vi "Core_Chem_User_Interface_v1.0.vi"() -> ()   [LabVIEW 2014]
uses:
  <vilib>/dex/Stream Element Allocation Mode.ctl
  C:/Program Files (x86)/National Instruments/LabVIEW 2014/examples/Data Communication/Network Streams/Simple Network Streams/support/Network Stream Command.ctl
  <vilib>/Platform/TimedLoop/XDataNode/timing_clust.ctl
  <vilib>/Platform/TimedLoop/XDataNode/nitl_modes.ctl
  <vilib>/Platform/TimedLoop/XDataNode/wakeup.ctl
  <vilib>/Utility/tcp.llb/UDP Multicast Read-Only Open.vi
  <vilib>/platform/TimedLoop/XDataNode/XDataNode.xnode
  <vilib>/Platform/TimedLoop/XDataNode/XDNodeRunTimeDep.lvlib
  <vilib>/FTP/NI_FTP.lvlib
panel:
  out "Create folder error out 2":errorcluster
  out "Network to cRIO live status":bool
  out "Create folder error out":errorcluster
  out "PRTUDP\nerror out":errorcluster
  in  "Confirm Flight Number":bool
  out "PRTAFT_UDP_In":string
  out "TWBOZO01":string
  out "CABOZO01":string
  out "TEIOZO01":string
  out "CHTSOO01":string
  out "CHFGGA01":string
  out "AL52CO01":string
  in  "Flight Number":string
  in  "Tab Control":T1(tab)
  out "MFM":dbl(graph)
  in  "name":string="239.1.4.6"
  in  "Port":u16=50001
  out "FGGA":string
  out "CO":string
  out "Ozone":string
  out "Cabin Ozone":string
  out "Ambient Ozone":string
  out "SO2":string
  out "CO Concentration":dbl(graph)
  out "Fluorsecence Cell Pressure":dbl(graph)
  out "Monochromater Flow":dbl(graph)
  out "Lamp Flow Controller":dbl(graph)
  in  "CO UDP Time Offset":i32=1
  out "CO2 Pressure\nDelivery (PSIA)":dbl(slide) scale=0.0..100.0
  out "CO CAL Status":bool
  out "Std\nContent (barG)":dbl(slide) scale=0.0..220.0
  out "N2\nContent (barG)":dbl(slide) scale=0.0..220.0
  out "CO2\nContent (barG)":dbl(slide) scale=0.0..170.0
  in  "CO CAL":bool
  in  "CO Vacuum (eV7)":bool
  out "CO Event error out":errorcluster
  out "CO command sender error out":errorcluster
  out "CO Zero":T2(array[cluster])
  out "CO Sensitivity":T3(array[cluster])
  in  "Ozone V6":bool
  out "TEI49C Sample Flow B":dbl(graph)
  out "TEi49C Concentration":dbl(graph)
  out "TEI49C Sample Flow A":dbl(graph)
  out "Ozone Event error out":errorcluster
  out "Ozone command sender error out":errorcluster
  out "Ozone Zeroing\nTime Remain (sec)":u32
  in  "Ozone Zeroing":bool
  in  "Ozone UDP Time Offset":i32=1
  in  "FGGA Pump":bool
  in  "FGGA Shutdown":bool
  in  "V1":bool
  in  "V2":bool
  in  "MFC_1\nSLPM Value":dbl
  in  "V3":bool
  in  "V4":bool
  in  "FGGA Restart":bool
  out "MFC1 Cal Flow":dbl(graph)
  out "Cell temperature":dbl(graph)
  out "Cell pressure":dbl(graph)
  out "CO2 Dry":dbl(graph)
  out "CH4 Dry":dbl(graph)
  out "H2O":dbl(graph)
  out "CO2":dbl(graph)
  out "CH4":dbl(graph)
  in  "Flush High Tank":bool
  in  "Flush Low Tank":bool
  in  "Flush Target Tank":bool
  out "Flush High Tank\nTime Remain (sec)":u32
  out "Flush Low Tank\nTime Remain (sec)":u32
  out "Flush Target Tank\nTime Remain (sec)":u32
  in  "High Cal":bool
  out "High Cal\nFlush Time Remain (sec)":u32
  out "High Cal\nCal Time Remain (sec)":u32
  in  "Low Cal":bool
  in  "Target Cal":bool
  in  "Span Cal":bool
  out "Low Cal\nFlush Time Remain (sec)":u32
  out "Low Cal\nCal Time Remain (sec)":u32
  out "Target Cal\nFlush Time Remain (sec)":u32
  out "Target Cal\nCal Time Remain (sec)":u32
  in  "MFC_1 User Set Value":dbl=3.0
  out "FGGA command sender error out":errorcluster
  out "FGGA Event Error out":errorcluster
  in  "FGGA UDP Time Offset":i32=1
  in  "FGGA pump\nsync to WoW":bool
  out "WoW Flag":string="0"
  in  "Inst_alm_thresh":i32=220
  in  "3hr_alm_thresh":i32=80
  in  "Simulate Inst Conc":i32
  in  "Simulate 3hr Average Conc":dbl
  in  "Simulate 2B Conc":bool
  out "2B Ozone concentration":dbl(graph)
  out "2B Ozone flow rate":dbl(graph)
  out "2BOzone Event error out":errorcluster
  out "2BOzone command sender error out":errorcluster
  in  "Ambient = OFF\nCabin = ON":bool
  in  "V9":bool
  in  "V8":bool
  in  "SO2 V6":bool
  in  "MFC_2\nSLPM Value":dbl
  in  "MFC_3\nSLPM Value":dbl=2.0
  in  "Simulate STEL Conc":dbl
  in  "Simulate TWA Conc":dbl
  in  "SO2 Offset":dbl
  in  "SO2 Slope":dbl=1.0
  in  "10mins STEL Limit":i32=700
  in  "8hr TWA Limit":i32=490
  in  "Simulate Conc":bool
  out "TEI43i MFC2 Cal Flow":dbl(graph)
  out "TEI43i MFC3 Sample Flow":dbl(graph)
  out "TEi43C Concentration":dbl(graph)
  out "TEI43C Sample Flow":dbl(graph)
  out "SO2 Event error out":errorcluster
  out "SO2 command sender error out":errorcluster
  in  "SO2 Flush":bool
  in  "SO2 CAL":bool
  in  "MFC_2 User Set Value":dbl=2.5
  in  "MFC_3 User Set Value":dbl=2.0
  out "SO2 Flush\nTime Remain (sec)":u32
  in  "SO2 Zeroing":bool
  out "SO2 Zeroing\nTime Remain (sec)":u32
  out "SO2 CAL\nTime Remain (sec)":u32
  in  "SO2 UDP Time Offset":i32=1
  in  "cRIO File IO Stop\n(USB Flash Drive Unmount)":bool
  in  "FTP ASCII Files to Local":bool
  in  "Transfer FGGA Files":bool
  out "File List":string[](array[string])
  out "FGGA File Transfer Error out":errorcluster
  out "Move to FM Error out":errorcluster
  out "USB Disk Space Used %":dbl(slide) scale=0.0..100.0
  out "PTP Sync":bool
  out "CPU Total %":dbl(graph)
  # "ch4\nco2\nh2o\npress_torr\ntemp_c\nfit_flag\nrda_usec\nrdb_usec\nch4_dry\nco2_dry\nMFC_1_absolute_pressure\nMFC_1_temperature\nMFC_1volumetic_flow\nMFC_1mass_flow\nMFC_1set_point\nV1\nV2\nV3\nV4\nrestart_FGGA\nFGGA_Pump\nCAL_MFC_1Set_Value"
  # "conc\ntemp\npress\nflow\nthreehr_oz\nInst_alarm\nthreehr_alarm"
  # "conc\ntemp\npress\nflow"
  # "concentration\npmt_volt\nlamp_volt\nlamp_intens\ninternal_temper\nreact_temper\nreact_press\nflow\nflags\nten_min_so2\neight_hr_so2\nten_min_so2_alm\neight_hr_so2_alm\nMFC_2absolute_pressure\nMFC_2temperature\nMFC_2volumetic_flow\nMFC_2mass_flow\nMFC_2set_point\nMFC_3_absolute_pressure\nMFC_3_temperature\nMFC_3volumetic_flow\nMFC_3mass_flow\nMFC_3set_point\nV6\nV8\nV9\nMFC2_Set_Value\nMFC3_Set_Value"
  # "conc\nbenchtemp\npress\ncellAint\ncellBint\nFlowA\nFlowB\nlamptemp\nflag\nV6"
  # "conc\ncounts\nsens\nzero\nlampflow\nlamptemp\nmonoflow\nmonotemp\nmonopress\ncellpress\ncalpress\ntemppmt\ncalconc\nerr\ncal_counter\nerr_counter\nCO_vacuum_status\nIn_Cal\nALEG1_press_delivery\nALREG1_press_content\nALREG2_press_content\nALREG3_press_content"
  # "DIRECT CONTROL"
  # "DIRECT CONTROLS"
  # "DIRECT CONTROLS"
  # "TEi43c"
  # "TEi43i"
  # "DIRECT CONTROLS"
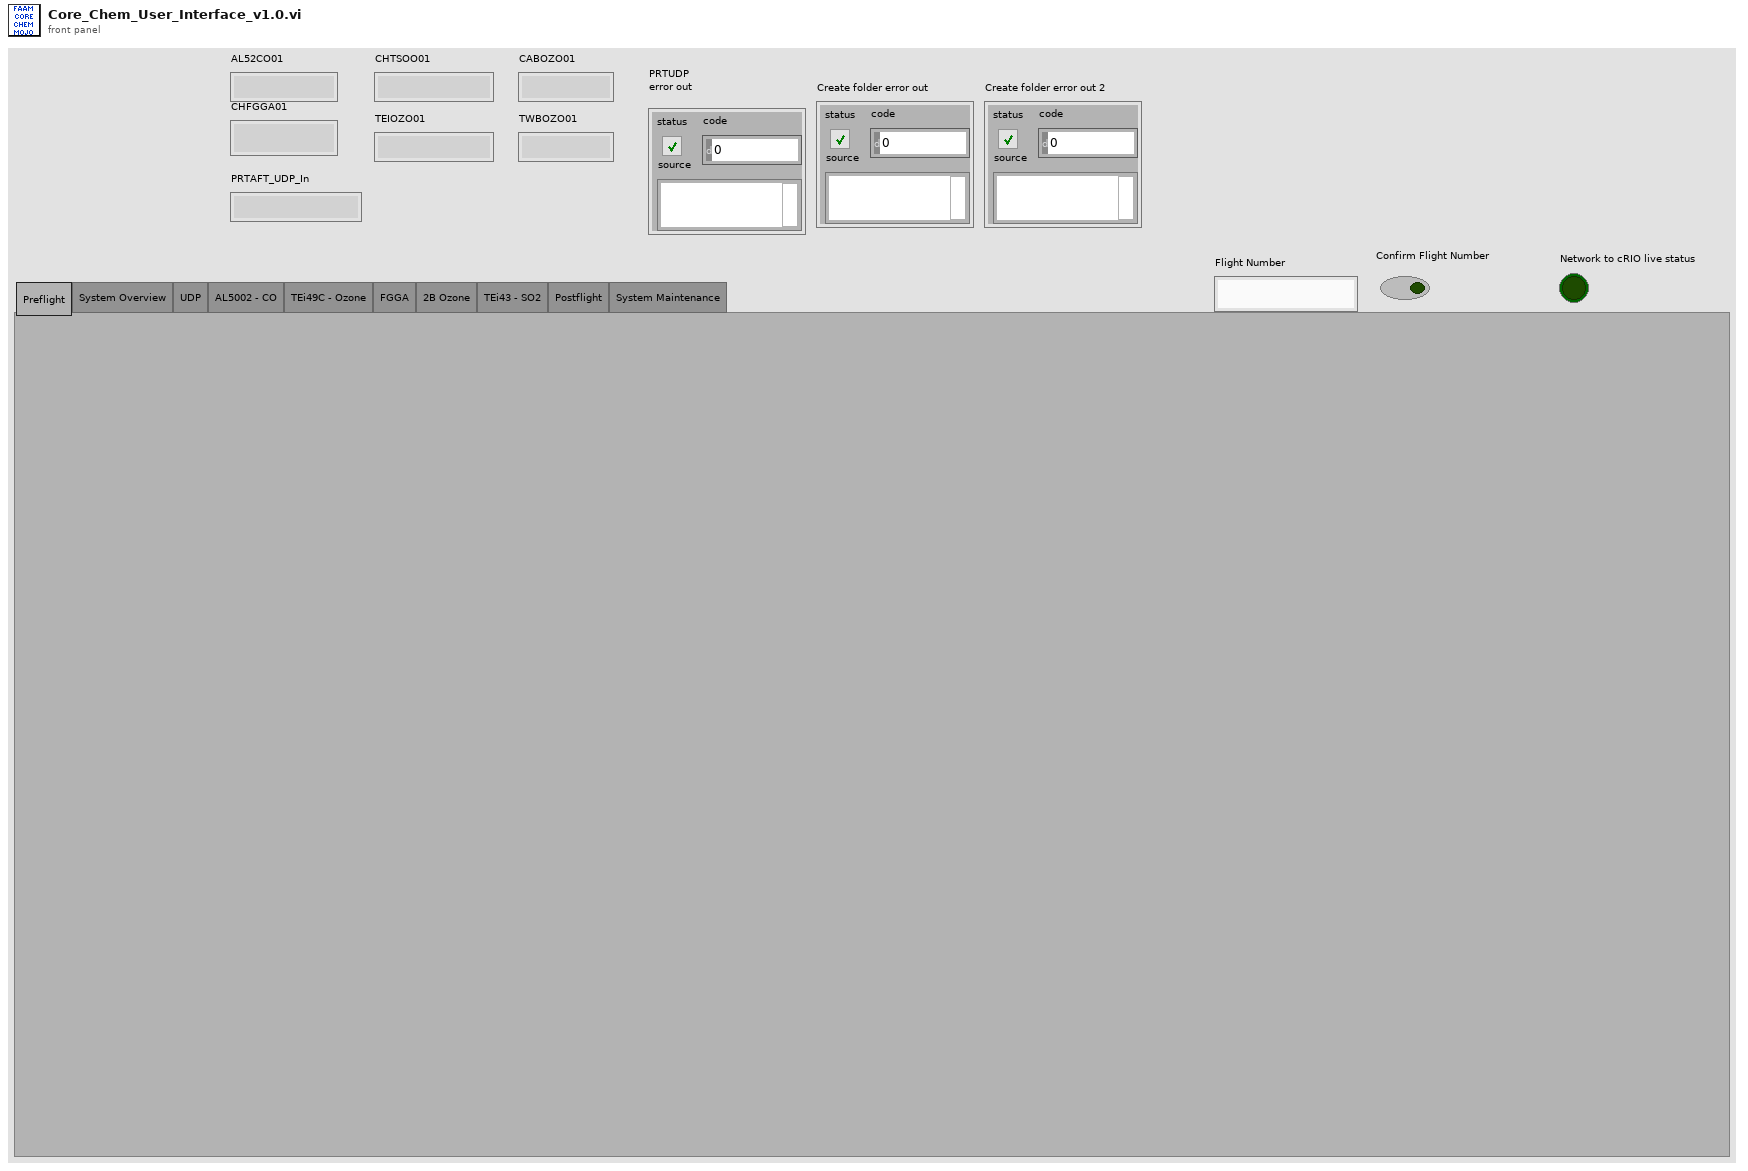
[diagram p1: front panel]
types:
  T1 = enum32{"Preflight", "System Overview", "UDP", "AL5002 - CO", "TEi49C - Ozone", "FGGA", "2B Ozone", "TEi43 - SO2", "Postflight", "System Maintenance"}
  T2 = cluster{"time stamp":timestamp, "CO Offset":dbl}[]
  T3 = cluster{"time stamp":timestamp, "CO Sensitivity":dbl}[]
  T4 = typedef "Network Stream Command.ctl" = cluster{"Message":string, "Message Data":variant}
  T5 = typedef "Stream Element Allocation Mode.ctl" = u32
  T6 = typedef "XDNodeRunTimeDep.lvlib/timing_clust.ctl" = cluster{"Expected End [f-1]":u64, "Actual End [f-1]":u64, "Finished Late? [f-1]":bool, "Expected End [i-1]":u64, "Actual End [i-1]":u64, "Finished Late? [i-1]":bool, "Expected Start [i]":u64, "Actual Start [i]":u64, "Expected Start [f]":u64, "Actual Start [f]":u64, "Source Name":string, "Structure Name":string, "Period":i64, "Deadline":i64, "Offset":i64, "Start":i64, "Priority":i32, "Timeout":i32, "Mode":T7, "Wakeup Reason":T8, "Error":errorcluster, "Source Type":string, "Secondary Source Type":string, "Global End Time":u64, "Global Start Time":u64, "Frame Duration":u64, "Iteration Duration":u64, "Assigned CPU":i32, "I/O Scan Engine Mode":u32}
  T7 = typedef "XDNodeRunTimeDep.lvlib/nitl_modes.ctl" = enum32{"No Change", "Process missed periods, maintain original phase", "Discard missed periods, maintain original phase", "Process missed periods, ignore original phase", "Discard missed periods, ignore original phase"}
  T8 = typedef "XDNodeRunTimeDep.lvlib/wakeup.ctl" = enum32{"Normal", "Aborted", "Asynchronous wakeup", "Timing source error", "Timed loop error", "Timeout"}
  T9 = typedef "NI_FTP.lvlib/FTP Session.ctl" = refnum<k5>
  T10 = typedef "NI_FTP.lvlib/FTP File Info.ctl" = cluster{"type":enum16{"unknown", "file", "dir", "link"}, "permissions":string, "owner":string, "group":string, "size":i32, "date":string, "name":string, "link name":string}
  T11 = cluster{"Message":string, "Message 2":string, "Message 3":string}
  T12 = cluster{"Message":string, "Message 2":string, "Message 3":string, "Message 4":string}
  T13 = cluster{"Message":string, "Message 3":string, "Message 4":string}
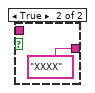
[diagram p7: hidden frame]
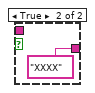
[diagram p8: hidden frame]
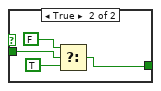
[diagram p9: hidden frame]
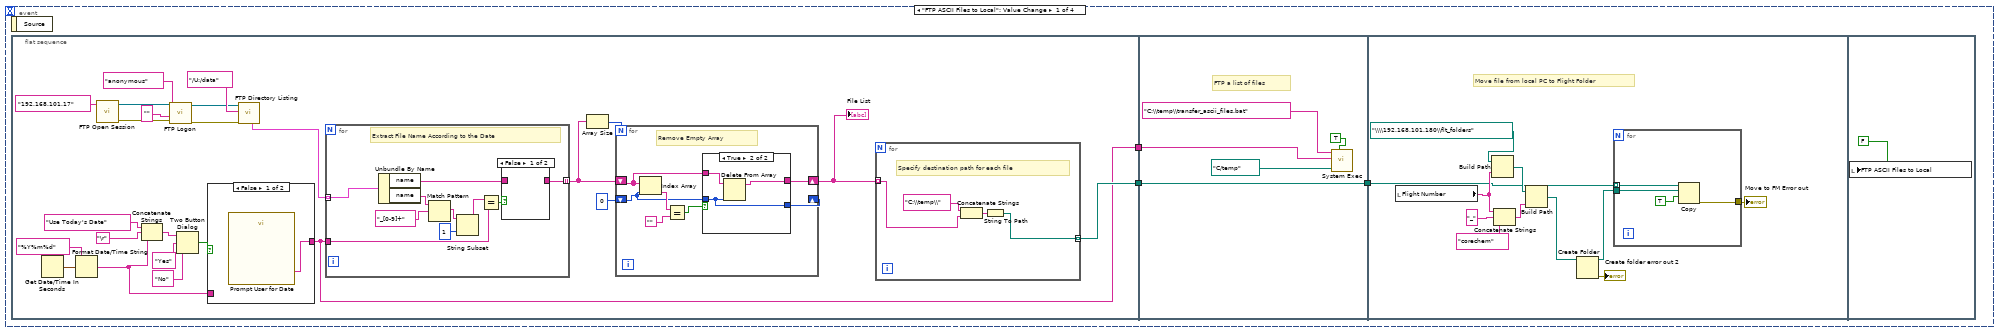
[diagram p12: hidden frame]
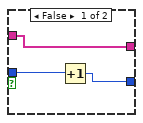
[diagram p14: hidden frame]
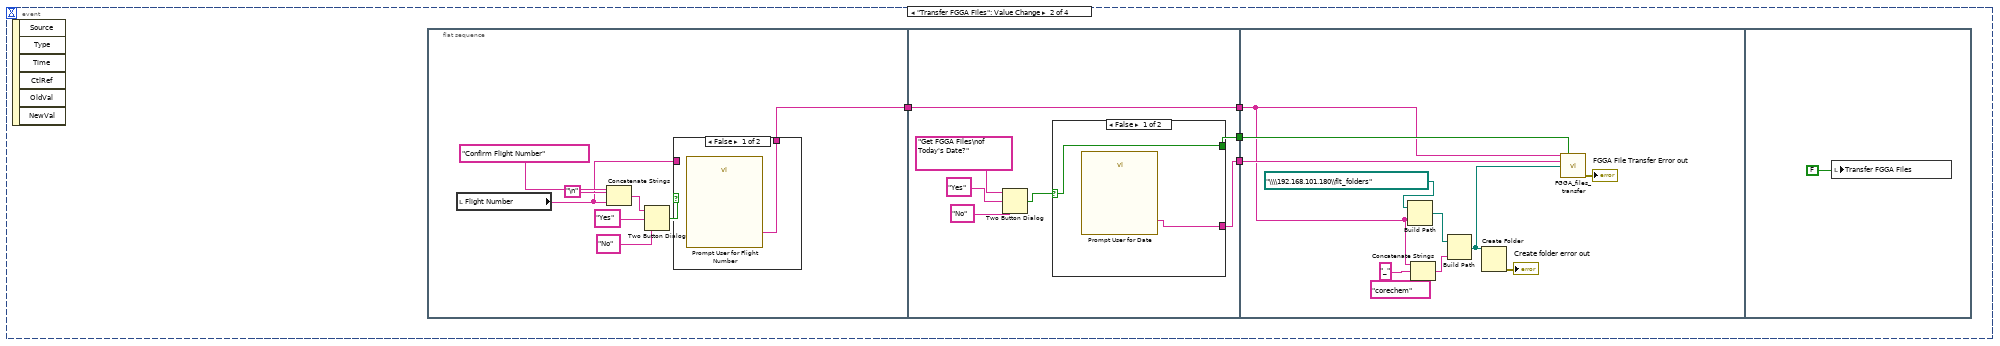
[diagram p16: hidden frame]
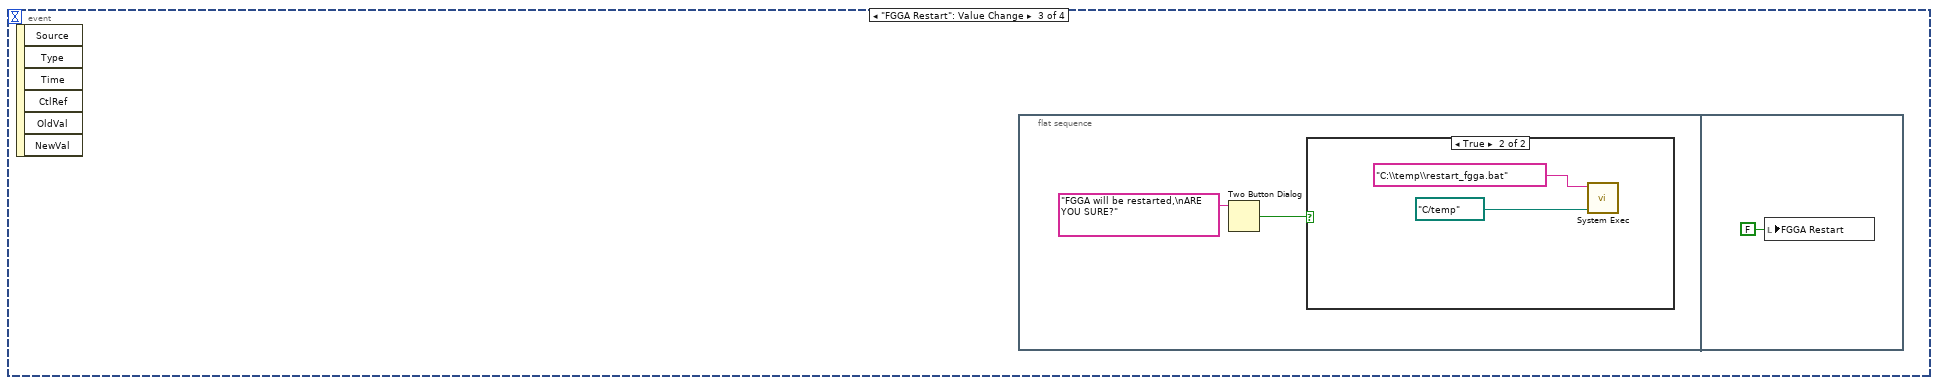
[diagram p19: hidden frame]
diagram:
  w4 = "XXXX"
  w7 = 0
  w8 = 0.0
  w14 = T4 {"Message"="", "Message Data"=variant} ("Message Cluster")
  w20 = T5 0 items=["allocate as needed", "pre-allocate"] ("element allocation mode")
  w26 = T4 {"Message"="", "Message Data"=variant} ("Message Cluster")
  w32 = T5 0 items=["allocate as needed", "pre-allocate"] ("element allocation mode")
  w37 = T4 {"Message"="", "Message Data"=variant} ("Message Cluster")
  w43 = T5 0 items=["allocate as needed", "pre-allocate"] ("element allocation mode")
  w53 = T5 0 items=["allocate as needed", "pre-allocate"] ("element allocation mode")
  w55 = T4 {"Message"="", "Message Data"=variant} ("Message Cluster")
  w62 = T5 0 items=["allocate as needed", "pre-allocate"] ("element allocation mode")
  w64 = T4 {"Message"="", "Message Data"=variant} ("Message Cluster")
  n1 = local write "cRIO File IO Stop\n(USB Flash Drive Unmount)"(FALSE ("Stop File Write")) -> ()
  n2 = local write "Flight Number"(w4) -> ()
  n3 = while {
    shift-right: [w68] -> _
    shift-left: w4 -> [w67]
    stop <- FALSE stop-if-true
    n4 = Not Equal?(x=w67, y="Flight Number") -> (x != y?=w70:bool)
    n5 = case shown="True" w70 {
      tunnel: [w73 w74] -> w68
      tunnel: "Flight Number" -> [_ w74]
      tunnel: w67 -> [w73 _]
      frame False {
      }
      frame True {
        n6 = One Button Dialog(message="Flight Number changed,\nPress flight number button to confirm") -> ()  [unwired: 1 in, 1 out]
      }
    }
    n7 = Wait (ms)(milliseconds to wait=u32 1000) -> ()  [unwired: 1 out]
  }
  n8 = while {
    stop <- w78 stop-if-true
    n9 = String To IP(1:"239.1.4.6" ("name")) -> (0:w85:u32)
    n10 = node-c288() -> (w87:T6)  [unwired: 4 in]
    n11 = call-poly <vilib>:"UDP Multicast Open.vi"("multicast addr"=w85, "port"=u16 50001) -> ("error out"=w81:errorcluster, "connection ID"=w82:refnum<k16>)  [unwired: 7 in, 1 out]
    n12 = timed-loop {
      tunnel: w82 -> [w99]
      tunnel: w81 -> [w98]
      timing: w87 -> [_]
      timing-out: [_] -> w86
      tunnel: [w92] -> w80
      tunnel: [w90] -> w79
      tunnel: [w88] -> w78
      stop <- w89 stop-if-true
      w88 = FALSE
      # "Extract string from port aft DLU"
      # "Get Flight Number loop"
      # "Read UDP & extract flight number and WoW flag"
      n13 = node-c288() -> ()  [unwired: 1 in, 1 out]
      n14 = UDP Read(connection ID=w99, 8:w98) -> (data out=w97:string, error out=w90:errorcluster, 3:w92:refnum<k16>)  [unwired: 2 in, 2 out]
      "PRTAFT_UDP_In" <- w97
      n15 = Match Pattern(string=w97, regular expression="$PRTAFT01") -> (after substring=w93:string)  [unwired: 1 in, 3 out]
      n16 = Not Equal?(x=w93, y="") -> (x != y?=w94:bool)
      n17 = case shown="True" w94 {
        tunnel: w93 -> [_ w112]
        frame False {
        }
        frame True {
          # "Extract flight number & WoW Flag"
          n18 = Spreadsheet String To Array(delimiter (Tab)=",", format string="%s", spreadsheet string=w112, array type (2D Dbl)=string[] []) -> (array=w106:string[])
          n19 = Index Array(array=w106, index=5) -> (element=w108:string)
          n20 = Index Array(array=w106, index=19) -> (element=w104:string)
          n21 = Equal?(x=w104, y="") -> (x = y?=w103:bool)
          n22 = Equal?(x=w108, y="") -> (x = y?=w111:bool)
          n23 = case shown="False" w111 {
            tunnel: [w119 "XXXX"] -> w109
            tunnel: w108 -> [w119 _]
            frame False {
            }
            frame True {
            }
          }
          n24 = case shown="False" w103 {
            tunnel: [w117 "XXXX"] -> w102
            tunnel: w104 -> [w117 _]
            frame False {
            }
            frame True {
            }
          }
          n25 = local write "Flight Number"(w109) -> ()
          n26 = local write "WoW Flag"(w102) -> ()
        }
      }
      n27 = Unbundle(w90) -> ("status"=w91:bool)  [unwired: 2 out]
      n28 = node-c288() -> ()  [unwired: 1 in, 1 out]
      n29 = Compound Arithmetic op=OR(w91, w88) -> (w89:bool)
    }
    n30 = Wait (ms)(milliseconds to wait=u32 1000) -> ()  [unwired: 1 out]
    n31 = node-c288(w86) -> ()  [unwired: 1 out]
    n32 = UDP Close(connection ID=w80, 8:w79) -> (error out=→"PRTUDP\nerror out":errorcluster)  [unwired: 1 out]
  }
  n33 = while {
    stop <- FALSE stop-if-true
    # "UDP Read"
    n34 = String To IP(1:"name") -> (0:w128:u32)
    n35 = call-poly <vilib>:"UDP Multicast Open.vi"("multicast addr"=w128, "port"="Port") -> ("error out"=w126:errorcluster, "connection ID"=w125:refnum<k16>)  [unwired: 7 in, 1 out]
    n36 = Wait (ms)(milliseconds to wait=u32 1000) -> ()  [unwired: 1 out]
    n37 = case shown="No Error" w126 {
      selector: w126 -> [w132 _]
      tunnel: w125 -> [w131 _]
      frame No Error {
        w130 = ""
        n38 = while {
          tunnel: w132 -> [w172]
          tunnel: w131 -> [w171]
          shift-right: [w167] -> _
          shift-left: w130 -> [w168]
          shift-right: [w158] -> _
          shift-left: w130 -> [w160]
          shift-right: [w152] -> _
          shift-left: w130 -> [w154]
          shift-right: [w146] -> _
          shift-left: w130 -> [w147]
          shift-right: [w140] -> _
          shift-left: w130 -> [w141]
          shift-right: [w133] -> _
          shift-left: w130 -> [w135]
          stop <- w170 stop-if-true
          n39 = UDP Read(connection ID=w171, 8:w172) -> (data out=w134:string, error out=w170:errorcluster)  [unwired: 2 in, 3 out]
          n40 = Match Pattern(string=w134, regular expression="$TEIOZO01,") -> (match substring=w166:string, after substring=w165:string)  [unwired: 1 in, 2 out]
          n41 = Match Pattern(string=w134, regular expression="$TWBOZO01,") -> (match substring=w144:string, after substring=w143:string)  [unwired: 1 in, 2 out]
          n42 = Match Pattern(string=w134, regular expression="$CABOZO01,") -> (match substring=w150:string, after substring=w149:string)  [unwired: 1 in, 2 out]
          n43 = Match Pattern(string=w134, regular expression="$CHTSOO01,") -> (match substring=w138:string, after substring=w137:string)  [unwired: 1 in, 2 out]
          n44 = Match Pattern(string=w134, regular expression="$CHFGGA01,") -> (match substring=w162:string, after substring=w161:string)  [unwired: 1 in, 2 out]
          n45 = Match Pattern(string=w134, regular expression="$AL52CO01,") -> (match substring=w156:string, after substring=w155:string)  [unwired: 1 in, 2 out]
          n46 = Concatenate Strings(w166, w165) -> (w164:string)
          n47 = Concatenate Strings(w144, w143) -> (w142:string)
          n48 = Concatenate Strings(w150, w149) -> (w148:string)
          n49 = Concatenate Strings(w138, w137) -> (w136:string)
          n50 = Concatenate Strings(w162, w161) -> (w159:string)
          n51 = Concatenate Strings(w156, w155) -> (w153:string)
          n52 = Replace Substring(4:w142, 5:w141) -> (1:w140:string)  [unwired: 2 in, 1 out]
          "TWBOZO01" <- w140
          n53 = Replace Substring(4:w164, 5:w168) -> (1:w167:string)  [unwired: 2 in, 1 out]
          "TEIOZO01" <- w167
          n54 = Replace Substring(4:w148, 5:w147) -> (1:w146:string)  [unwired: 2 in, 1 out]
          "CABOZO01" <- w146
          n55 = Replace Substring(4:w136, 5:w135) -> (1:w133:string)  [unwired: 2 in, 1 out]
          "CHTSOO01" <- w133
          n56 = Replace Substring(4:w153, 5:w154) -> (1:w152:string)  [unwired: 2 in, 1 out]
          "AL52CO01" <- w152
          n57 = Replace Substring(4:w159, 5:w160) -> (1:w158:string)  [unwired: 2 in, 1 out]
          "CHFGGA01" <- w158
        }
      }
      frame Error {
      }
    }
  }
  n58 = Obtain Queue(name (unnamed)="CO_Command", element data type=w64) -> (queue out=w13:refnum<queue>, error out=w58:errorcluster)  [unwired: 3 in, 1 out]
  n59 = Create Network Stream Writer Endpoint(6:w62, 7:10 ("writer buffer size"), 9:w64, 10:"//192.168.101.17/command/reader/CO" ("reader url"), 11:"/command/writer/CO" ("writer name")) -> (0:w61:errorcluster, 3:w60:refnum<k21>)  [unwired: 2 in]
  n60 = while {
    tunnel: w13 -> [w176]
    tunnel: w58 -> [w175]
    tunnel: [w173] -> _
    stop <- FALSE stop-if-true
    # "CO UI Event Handler Loop"
    n61 = event shown="[4] \"Confirm Flight Number\": Value Change" {
      selector: _ -> [_ _ _ _ _]
      dyn-events: _ -> [_ _ _ _ _]
      timeout: _ -> [_ _ _ _ _]
      tunnel: w176 -> [w183 w190 w194 w201 w208]
      tunnel: w175 -> [w182 w189 w193 w200 w207]
      tunnel: [w177 w184 w192 w199 w206] -> w173
      event "CO CAL": Value Change {
        n62 = event-data() -> ("NewVal"=w180:bool)  [unwired: 1 in]
        n63 = Bundle(cluster=T4 {"Message"="", "Message Data"=variant} ("Message Cluster"), "Message"="CO CAL", "Message Data"=w180) -> (w178:T4)
        n64 = Enqueue Element(queue=w183, element=w178, error in (no error)=w182) -> (error out=w177:errorcluster)  [unwired: 1 in, 2 out]
      }
      event "CO UDP Time Offset": Value Change {
        n65 = event-data() -> ("NewVal"=w187:i32)  [unwired: 1 in]
        n66 = Bundle(cluster=T4 {"Message"="", "Message Data"=variant} ("Message Cluster"), "Message"="UDP Time Offset", "Message Data"=w187) -> (w185:T4)
        n67 = Enqueue Element(queue=w190, element=w185, error in (no error)=w189) -> (error out=w184:errorcluster)  [unwired: 1 in, 2 out]
      }
      event "CO Vacuum (eV7)": Value Change {
        n68 = event-data() -> ("NewVal"=w191:bool)  [unwired: 1 in]
        n69 = Bundle(cluster=T4 {"Message"="", "Message Data"=variant} ("Message Cluster"), "Message"="CO Vacuum", "Message Data"=w191) -> (w195:T4)
        n70 = Enqueue Element(queue=w194, element=w195, error in (no error)=w193) -> (error out=w192:errorcluster)  [unwired: 1 in, 2 out]
      }
      event "cRIO File IO Stop\n(USB Flash Drive Unmount)": Value Change {
        n71 = event-data() -> ("NewVal"=w198:bool)  [unwired: 1 in]
        n72 = Bundle(cluster=T4 {"Message"="", "Message Data"=variant} ("Message Cluster"), "Message"="Stop File Write", "Message Data"=w198) -> (w202:T4)
        n73 = Enqueue Element(queue=w201, element=w202, error in (no error)=w200) -> (error out=w199:errorcluster)  [unwired: 1 in, 2 out]
      }
      event "Confirm Flight Number": Value Change {
        n74 = event-data() -> ()  [unwired: 1 in, 1 out]
        n75 = local read "Flight Number"() -> (w205:string)
        n76 = Bundle(cluster=T4 {"Message"="", "Message Data"=variant} ("Message Cluster"), "Message"="Flight Number", "Message Data"=w205) -> (w209:T4)
        n77 = Enqueue Element(queue=w208, element=w209, error in (no error)=w207) -> (error out=w206:errorcluster)  [unwired: 1 in, 2 out]
      }
    }
    "CO Event error out" <- w173
  }
  n78 = while {
    tunnel: w13 -> [w219]
    shift-right: [w214] -> _
    shift-left: w60 -> [w216]
    shift-right: [w212] -> w49
    shift-left: w61 -> [w218]
    tunnel: w58 -> [w213]
    stop <- w212 stop-if-true
    # "CO UI Command Sender"
    n79 = Dequeue Element(queue=w219, error in (no error)=w213) -> (element=w215:T4)  [unwired: 1 in, 3 out]
    n80 = Unbundle By Name(w215) -> ("Message"=w217:string)
    n81 = case shown="\"UDP Time Offset\"" w217 {
      tunnel: w218 -> [w220 w224 w231 w238 w245 w252]
      tunnel: w216 -> [w221 w227 w234 w241 w248 w255]
      tunnel: w215 -> [_ w226 w233 w240 w247 w254]
      tunnel: [w220 w223 w230 w237 w244 w251] -> w212
      tunnel: [w221 w222 w229 w236 w243 w250] -> w214
      frame "False", Default {
      }
      frame "CO CAL" {
        n82 = shared-variable-write(w227, w224, w226) -> (w225:refnum<k21>, w228:errorcluster)  [unwired: 1 in, 1 out]
        n83 = Flush Stream(8:w228, 11:w225) -> (0:w223:errorcluster, 3:w222:refnum<k21>)  [unwired: 2 in, 1 out]
      }
      frame "UDP Time Offset" {
        n84 = shared-variable-write(w234, w231, w233) -> (w232:refnum<k21>, w235:errorcluster)  [unwired: 1 in, 1 out]
        n85 = Flush Stream(8:w235, 11:w232) -> (0:w230:errorcluster, 3:w229:refnum<k21>)  [unwired: 2 in, 1 out]
      }
      frame "Stop File Write" {
        n86 = shared-variable-write(w241, w238, w240) -> (w239:refnum<k21>, w242:errorcluster)  [unwired: 1 in, 1 out]
        n87 = Flush Stream(8:w242, 11:w239) -> (0:w237:errorcluster, 3:w236:refnum<k21>)  [unwired: 2 in, 1 out]
      }
      frame "Flight Number" {
        n88 = shared-variable-write(w248, w245, w247) -> (w246:refnum<k21>, w249:errorcluster)  [unwired: 1 in, 1 out]
        n89 = Flush Stream(8:w249, 11:w246) -> (0:w244:errorcluster, 3:w243:refnum<k21>)  [unwired: 2 in, 1 out]
      }
      frame "CO Vacuum" {
        n90 = shared-variable-write(w255, w252, w254) -> (w253:refnum<k21>, w256:errorcluster)  [unwired: 1 in, 1 out]
        n91 = Flush Stream(8:w256, 11:w253) -> (0:w251:errorcluster, 3:w250:refnum<k21>)  [unwired: 2 in, 1 out]
      }
    }
  }
  "CO command sender error out" <- w49
  n92 = node-c288() -> (w12:T6)  [unwired: 4 in]
  n93 = Initialize Array(cluster{"time stamp":timestamp, "Y":dbl} {"time stamp"=timestamp(0 s since 1904-01-01), "Y"=0.0}, 30 ("dimension size")) -> (w9:cluster{"time stamp":timestamp, "Y":dbl}[])
  n94 = timed-loop {
    timing: w12 -> [_]
    timing-out: [_] -> w11
    stop <- _ stop-if-true
    # "PC Tasks"
    n95 = node-c288() -> ()  [unwired: 1 in, 1 out]
    n96 = event shown="[3] \"FGGA Shutdown\": Value Change" {
      selector: _ -> [_ _ _ _]
      dyn-events: _ -> [_ _ _ _]
      timeout: _ -> [_ _ _ _]
      event "FTP ASCII Files to Local": Value Change {
        n97 = event-data() -> ()  [unwired: 1 in, 1 out]
        n98 = flat-sequence {
          tunnel: [w263] -> w261
          tunnel: [w262] -> w259
          tunnel: w261 -> [w320]
          tunnel: [w320] -> w260
          tunnel: w259 -> [w316]
          tunnel: w260 -> [w325]
          frame #0 {
            n99 = Get Date/Time In Seconds() -> (seconds since 1Jan1904=w267:timestamp)
            n100 = Format Date/Time String(time format string (%c)="%Y%m%d", seconds (now)=w267) -> (date/time string=w265:string)  [unwired: 1 in]
            n101 = call <vilib>:"FTP Open Session.vi"("address"="192.168.101.17") -> ("error out"=w282:errorcluster, "ftp session"=w283:T9)  [unwired: 7 in, 2 out]
            n102 = Concatenate Strings("Use Today's Date" ("message"), "\r", w265) -> (w271:string)
            n103 = call <vilib>:"FTP Logon.vi"("error in (no error)"=w282, "password"="", "user"="anonymous", "ftp session"=w283) -> ("error out"=w279:errorcluster, "ftp session out"=w278:T9)  [unwired: 4 in, 2 out]
            n104 = Two Button Dialog(message=w271, 1:"No" ("F button name (\"Cancel\")"), 2:"Yes" ("T button name (\"OK\")")) -> (T button?=w268:bool)
            n105 = case shown="False" w268 {
              tunnel: [w286 w287] -> w262
              tunnel: w265 -> [_ w287]
              frame False {
                n106 = call "Prompt User for Date"() -> ("Date"=w286:string)  [unwired: 17 in, 2 out]
              }
              frame True {
              }
            }
            n107 = call <vilib>:"FTP Directory Listing.vi"("error in (no error)"=w279, "directory path"="/U:/data", "ftp session"=w278) -> ("dir list"=w277:T10[])  [unwired: 4 in, 4 out]
            n108 = for {
              tunnel: w277 -> [w307] mode=indexing
              tunnel: [w306] -> w274 mode=indexing
              tunnel: w262 -> [w305]
              # "Extract File Name According to the Date"
              n109 = Unbundle By Name(w307) -> ("name"=w313:string, "name"=w312:string)
              n110 = Match Pattern(string=w312, regular expression="_[0-9]+") -> (match substring=w310:string)  [unwired: 1 in, 3 out]
              n111 = String Subset(string=w310, offset (0)=1) -> (substring=w308:string)  [unwired: 1 in]
              n112 = Equal?(x=w308, y=w305) -> (x = y?=w314:bool)
              n113 = case shown="False" w314 {
                tunnel: w313 -> [_ w315]
                tunnel: [_ w315] -> w306
                frame False {
                }
                frame True {
                }
              }
            }
            n114 = Array Size(array=w274) -> (size(s)=w276:i32)
            n115 = for {
              N: w276 -> [_]
              shift-right: [w294] -> w264
              shift-left: w274 -> [w295]
              shift-right: [w292] -> _
              shift-left: 0 -> [w293]
              # "Remove Empty Array"
              n116 = Index Array(array=w295, index=w293) -> (element=w297:string)
              n117 = Equal?(x=w297, y="") -> (x = y?=w296:bool)
              n118 = case shown="True" w296 {
                tunnel: w295 -> [w301 w304]
                tunnel: w293 -> [w300 w302]
                tunnel: [w301 w303] -> w294
                tunnel: [w299 w302] -> w292
                frame False {
                  n119 = Increment(x=w300) -> (x+1=w299:i32)
                }
                frame True {
                  n120 = Delete From Array(array=w304, index=w302) -> (array with subset deleted=w303:string[])  [unwired: 1 in, 1 out]
                }
              }
            }
            "File List" <- w264
            n121 = for {
              tunnel: w264 -> [w290] mode=indexing
              tunnel: [w288] -> w263 mode=indexing
              # "Specify destination path for each file"
              n122 = Concatenate Strings("C:\\temp\\", w290) -> (w289:string)
              n123 = String To Path(string=w289) -> (path=w288:path)
            }
          }
          frame #1 {
            # "FTP a list of files"
            n124 = call <vilib>:"System Exec.vi"("wait until completion? (T)"=TRUE, "working directory"=path "C:/temp", "standard input"=w316, "command line"="C:\\temp\\transfer_ascii_files.bat") -> ()  [unwired: 4 in, 4 out]
          }
          frame #2 {
            # "Move file from local PC to Flight Folder"
            n125 = local read "Flight Number"() -> (w326:string)
            n126 = Build Path(base path=path "\\\\192.168.101.180\\flt_folders" ("path"), name or relative path=w326) -> (appended path=w328:path)
            n127 = Concatenate Strings(w326, "_" ("string"), "corechem" ("string")) -> (w327:string)
            n128 = Build Path(base path=w328, name or relative path=w327) -> (appended path=w322:path)
            n129 = Create Folder(path (use dialog)=w322) -> (created path=w321:path, error out=→"Create folder error out 2":errorcluster)  [unwired: 2 in, 1 out]
            n130 = for {
              tunnel: w321 -> [w335]
              tunnel: [w334] -> w324
              tunnel: w325 -> [w332] mode=indexing
              n131 = Copy(9:TRUE ("overwrite (F)"), 10:w335, 11:w332) -> (0:w334:errorcluster)  [unwired: 2 in, 2 out]
            }
            "Move to FM Error out" <- w324
          }
          frame #3 {
            n132 = local write "FTP ASCII Files to Local"(FALSE ("FTP Files to Local")) -> ()
          }
        }
      }
      event "Transfer FGGA Files": Value Change {
        n133 = event-data() -> ()  [unwired: 1 in, 6 out]
        n134 = flat-sequence {
          tunnel: [w341] -> w340
          tunnel: w340 -> [w353]
          tunnel: [w353] -> w339
          tunnel: [w352] -> w338
          tunnel: [w351] -> w337
          tunnel: w339 -> [w369]
          tunnel: w338 -> [w371]
          tunnel: w337 -> [w370]
          frame #0 {
            n135 = local read "Flight Number"() -> (w342:string)
            n136 = Concatenate Strings("Confirm Flight Number" ("message"), "\n", w342) -> (w344:string)
            n137 = Two Button Dialog(message=w344, 1:"No" ("F button name (\"Cancel\")"), 2:"Yes" ("T button name (\"OK\")")) -> (T button?=w348:bool)
            n138 = case shown="False" w348 {
              tunnel: w342 -> [_ w350]
              tunnel: [w349 w350] -> w341
              frame False {
                n139 = call "Prompt User for Flight Number"() -> ("Flight Number BXXX"=w349:string)  [unwired: 17 in, 2 out]
              }
              frame True {
              }
            }
          }
          frame #1 {
            n140 = Two Button Dialog(message="Get FGGA Files\nof Today's Date?", 1:"No" ("F button name (\"Cancel\")"), 2:"Yes" ("T button name (\"OK\")")) -> (T button?=w357:bool)
            n141 = case shown="False" w357 {
              selector: w357 -> [w359 w360]
              tunnel: [w359 w360] -> w351
              tunnel: [w358 _] -> w352
              frame False {
                n142 = call "Prompt User for Date"() -> ("Date"=w358:string)  [unwired: 17 in, 2 out]
              }
              frame True {
              }
            }
          }
          frame #2 {
            n143 = Build Path(base path=path "\\\\192.168.101.180\\flt_folders" ("path"), name or relative path=w369) -> (appended path=w363:path)
            n144 = Concatenate Strings(w369, "_" ("string"), "corechem" ("string")) -> (w362:string)
            n145 = Build Path(base path=w363, name or relative path=w362) -> (appended path=w368:path)
            n146 = Create Folder(path (use dialog)=w368) -> (error out=→"Create folder error out":errorcluster)  [unwired: 2 in, 2 out]
            n147 = call "FGGA_files_transfer.vi"("Flight_num"=w369, "Get current?"=w370, "Date"=w371, "Flight Folder Path"=w368) -> ("error IO"=→"FGGA File Transfer Error out":errorcluster)  [unwired: 11 in]
          }
          frame #3 {
            n148 = local write "Transfer FGGA Files"(FALSE) -> ()
          }
        }
      }
      event "FGGA Restart": Value Change {
        n149 = event-data() -> ()  [unwired: 1 in, 6 out]
        n150 = flat-sequence {
          frame #0 {
            n151 = Two Button Dialog(message="FGGA will be restarted,\nARE YOU SURE?") -> (T button?=w374:bool)  [unwired: 2 in]
            n152 = case shown="True" w374 {
              frame False {
              }
              frame True {
                n153 = call <vilib>:"System Exec.vi"("working directory"=path "C:/temp", "command line"="C:\\temp\\restart_fgga.bat") -> ()  [unwired: 6 in, 4 out]
              }
            }
          }
          frame #1 {
            n154 = local write "FGGA Restart"(FALSE ("FGGA Restart")) -> ()
          }
        }
      }
      event "FGGA Shutdown": Value Change {
        n155 = event-data() -> ()  [unwired: 1 in, 6 out]
        n156 = flat-sequence {
          frame #0 {
            n157 = Two Button Dialog(message="FGGA will be shutdown,\nARE YOU SURE?") -> (T button?=w379:bool)  [unwired: 2 in]
            n158 = case shown="True" w379 {
              frame False {
              }
              frame True {
                n159 = call <vilib>:"System Exec.vi"("working directory"=path "C:/temp", "command line"="C:\\temp\\shutdown_fgga.bat") -> ()  [unwired: 6 in, 4 out]
              }
            }
          }
          frame #1 {
            n160 = local write "FGGA Shutdown"(FALSE ("FGGA Restart")) -> ()
          }
        }
      }
    }
    n161 = node-c288() -> ()  [unwired: 1 in, 1 out]
  }
  n162 = while {
    shift-right: [w446] -> _
    shift-left: w8 -> [w444]
    shift-right: [w448] -> _
    shift-left: w7 -> [w449]
    shift-right: [w447] -> _
    shift-left: w9 -> [w451]
    shift-right: [w439] -> _
    shift-left: w9 -> [w441]
    shift-right: [w436] -> _
    shift-left: w8 -> [w435]
    shift-right: [w438] -> _
    shift-left: w7 -> [w440]
    shift-right: [w431] -> _
    shift-left: FALSE -> [w432]
    stop <- FALSE stop-if-true
    w570 = "%s" ("format string")
    w575 = "%s" ("format string")
    w580 = "%s" ("format string")
    w586 = "%s" ("format string")
    w592 = "%s" ("format string")
    w596 = "%s" ("format string")
    # "UDP Data Processing"
    n163 = local read "CHFGGA01"() -> (w599:string)
    n164 = local read "TWBOZO01"() -> (w574:string)
    n165 = local read "AL52CO01"() -> (w591:string)
    n166 = local read "CABOZO01"() -> (w579:string)
    n167 = local read "TEIOZO01"() -> (w585:string)
    n168 = local read "CHTSOO01"() -> (w569:string)
    n169 = local read "Ambient = OFF\nCabin = ON"() -> (w473:bool)
    n170 = Spreadsheet String To Array(delimiter (Tab)=",", format string=w596, spreadsheet string=w599, array type (2D Dbl)=string[] []) -> (array=w546:string[])
    n171 = Spreadsheet String To Array(delimiter (Tab)=",", format string=w592, spreadsheet string=w591, array type (2D Dbl)=string[] []) -> (array=w567:string[])
    n172 = Spreadsheet String To Array(delimiter (Tab)=",", format string=w580, spreadsheet string=w579, array type (2D Dbl)=string[] []) -> (array=w470:string[])
    n173 = Spreadsheet String To Array(delimiter (Tab)=",", format string=w586, spreadsheet string=w585, array type (2D Dbl)=string[] []) -> (array=w544:string[])
    n174 = Spreadsheet String To Array(delimiter (Tab)=",", format string=w575, spreadsheet string=w574, array type (2D Dbl)=string[] []) -> (array=w469:string[])
    n175 = Spreadsheet String To Array(delimiter (Tab)=",", format string=w570, spreadsheet string=w569, array type (2D Dbl)=string[] []) -> (array=w542:string[])
    n176 = Array To Spreadsheet String(delimiter (Tab)="\r", array=w546, 3:w596) -> (spreadsheet string=→"FGGA":string)
    n177 = Array To Spreadsheet String(delimiter (Tab)="\r", array=w567, 3:w592) -> (spreadsheet string=→"CO":string)
    n178 = Array To Spreadsheet String(delimiter (Tab)="\r", array=w470, 3:w580) -> (spreadsheet string=→"Cabin Ozone":string)
    n179 = Array To Spreadsheet String(delimiter (Tab)="\r", array=w544, 3:w586) -> (spreadsheet string=→"Ozone":string)
    n180 = Array To Spreadsheet String(delimiter (Tab)="\r", array=w469, 3:w575) -> (spreadsheet string=→"Ambient Ozone":string)
    n181 = Array To Spreadsheet String(delimiter (Tab)="\r", array=w542, 3:w570) -> (spreadsheet string=→"SO2":string)
    n182 = Select(t=w470, s=w473, f=w469) -> (s? t:f=w468:string[])
    n183 = Index Array(array=w542, index #1=6 ("index"), index #2=4 ("index"), index #3=3 ("index"), index #4=7 ("index"), index #5=8 ("index"), index #6=15 ("index"), index #7=24 ("index"), index #8=29 ("index")) -> (element #1=w459:string, element #2=w525:string, element #3=w520:string, element #4=w513:string, element #5=w489:string, element #6=w488:string, element #7=w396:string, element #8=w395:string)
    n184 = Index Array(array=w468, index #1=8 ("index"), index #2=11 ("index")) -> (element #1=w462:string, element #2=w463:string)
    n185 = Index Array(array=w544, index #1=6 ("index"), index #2=4 ("index"), index #3=3 ("index"), index #4=7 ("index"), index #5=9 ("index"), index #6=14 ("index"), index #7=15 ("index")) -> (element #1=w538:string, element #2=w526:string, element #3=w521:string, element #4=w506:string, element #5=w479:string, element #6=w478:string, element #7=w477:string)
    n186 = Scan Value(string=w462, format string="%f") -> (value=→"2B Ozone concentration":dbl)  [unwired: 1 in, 1 out]
    n187 = Scan Value(string=w463, format string="%f") -> (value=→"2B Ozone flow rate":dbl)  [unwired: 1 in, 1 out]
    n188 = Scan Value(string=w396, format string="%f") -> (value=→"TEI43i MFC2 Cal Flow":dbl)  [unwired: 1 in, 1 out]
    n189 = Scan Value(string=w395, format string="%f") -> (value=→"TEI43i MFC3 Sample Flow":dbl)  [unwired: 1 in, 1 out]
    n190 = Scan Value(string=w489, format string="%f") -> (value=→"TEi43C Concentration":dbl)  [unwired: 1 in, 1 out]
    n191 = Scan Value(string=w488, format string="%f") -> (value=→"TEI43C Sample Flow":dbl)  [unwired: 1 in, 1 out]
    n192 = Index Array(array=w546, index #1=6 ("index"), index #2=4 ("index"), index #3=3 ("index"), index #4=7 ("index"), index #5=8 ("index"), index #6=9 ("index"), index #7=10 ("index"), index #8=16 ("index"), index #9=17 ("index"), index #10=11 ("index"), index #11=12 ("index"), index #12=21 ("index")) -> (element #1=w540:string, element #2=w528:string, element #3=w523:string, element #4=w508:string, element #5=w420:string, element #6=w417:string, element #7=w412:string, element #8=w410:string, element #9=w407:string, element #10=w402:string, element #11=w401:string, element #12=w388:string)
    n193 = Index Array(array=w567, index #1=2 ("index"), index #2=27 ("index"), index #3=28 ("index"), index #4=29 ("index"), index #5=30 ("index"), index #6=31 ("index"), index #7=6 ("index"), index #8=4 ("index"), index #9=3 ("index"), index #10=8 ("index"), index #11=14 ("index"), index #12=16 ("index"), index #13=19 ("index"), index #14=12 ("index"), index #15=13 ("index"), index #16=10 ("index")) -> (element #1=w430:string, element #2=w510:string, element #3=w557:string, element #4=w551:string, element #5=w549:string, element #6=w550:string, element #7=w539:string, element #8=w527:string, element #9=w522:string, element #10=w511:string, element #11=w498:string, element #12=w495:string, element #13=w494:string, element #14=w454:string, element #15=w453:string, element #16=w384:string)
    n194 = Decimal String To Number(string=w430) -> (number=w428:i32)  [unwired: 2 in, 1 out]
    n195 = call "Find_Data_SubVI.vi"("FGGA"=w540, "CO"=w539, "Ozone"=w538, "SO2"=w459) -> ("Output Value"=→"CPU Total %":dbl)  [unwired: 11 in]
    n196 = call "Find_Data_SubVI.vi"("FGGA"=w528, "CO"=w527, "Ozone"=w526, "SO2"=w525) -> ("Output Value"=→"MFM":dbl)  [unwired: 11 in]
    n197 = call "Find_Data_SubVI.vi"("FGGA"=w523, "CO"=w522, "Ozone"=w521, "SO2"=w520) -> ("Output Value"=w519:dbl)  [unwired: 11 in]
    n198 = call "Find_Data_SubVI.vi"("FGGA"=w508, "CO"=w511, "Ozone"=w506, "SO2"=w513) -> ("Output Value"=→"USB Disk Space Used %":dbl)  [unwired: 11 in]
    n199 = Not Equal To 0?(x=w519) -> (x != 0?=→"PTP Sync":bool)
    n200 = Add(x=w428, y=u32 2082844800) -> (x+y=w427:u32)
    n201 = Scan Value(string=w388, format string="%f") -> (value=→"MFC1 Cal Flow":dbl)  [unwired: 1 in, 1 out]
    n202 = Scan Value(string=w401, format string="%f") -> (value=→"Cell temperature":dbl)  [unwired: 1 in, 1 out]
    n203 = Scan Value(string=w402, format string="%f") -> (value=→"Cell pressure":dbl)  [unwired: 1 in, 1 out]
    n204 = Scan Value(string=w407, format string="%f") -> (value=→"CH4 Dry":dbl)  [unwired: 1 in, 1 out]
    n205 = Scan Value(string=w410, format string="%f") -> (value=→"CO2 Dry":dbl)  [unwired: 1 in, 1 out]
    n206 = Scan Value(string=w412, format string="%f") -> (value=→"H2O":dbl)  [unwired: 1 in, 1 out]
    n207 = Scan Value(string=w417, format string="%f") -> (value=→"CO2":dbl)  [unwired: 1 in, 1 out]
    n208 = Scan Value(string=w420, format string="%f") -> (value=→"CH4":dbl)  [unwired: 1 in, 1 out]
    n209 = Scan Value(string=w550, format string="%f") -> (value=→"Std\nContent (barG)":dbl)  [unwired: 1 in, 1 out]
    n210 = Scan Value(string=w510, format string="%d", default (0 dbl)=u32 0) -> (value=w564:u32)  [unwired: 1 out]
    n211 = Scan Value(string=w549, format string="%f") -> (value=→"N2\nContent (barG)":dbl)  [unwired: 1 in, 1 out]
    n212 = Scan Value(string=w551, format string="%f") -> (value=→"CO2\nContent (barG)":dbl)  [unwired: 1 in, 1 out]
    n213 = Scan Value(string=w557, format string="%f") -> (value=→"CO2 Pressure\nDelivery (PSIA)":dbl)  [unwired: 1 in, 1 out]
    n214 = To Time Stamp(1:w427) -> (0:w434:timestamp)
    n215 = Scan Value(string=w479, format string="%f") -> (value=→"TEi49C Concentration":dbl)  [unwired: 1 in, 1 out]
    n216 = Scan Value(string=w478, format string="%f") -> (value=→"TEI49C Sample Flow A":dbl)  [unwired: 1 in, 1 out]
    n217 = Scan Value(string=w498, format string="%f") -> (value=→"Lamp Flow Controller":dbl)  [unwired: 1 in, 1 out]
    n218 = Scan Value(string=w384, format string="%f") -> (value=→"CO Concentration":dbl)  [unwired: 1 in, 1 out]
    n219 = Scan Value(string=w477, format string="%f") -> (value=→"TEI49C Sample Flow B":dbl)  [unwired: 1 in, 1 out]
    n220 = Scan Value(string=w495, format string="%f") -> (value=→"Monochromater Flow":dbl)  [unwired: 1 in, 1 out]
    n221 = Scan Value(string=w494, format string="%f") -> (value=→"Fluorsecence Cell Pressure":dbl)  [unwired: 1 in, 1 out]
    n222 = Not Equal To 0?(x=w564) -> (x != 0?=→"CO CAL Status":bool)
    n223 = call "ping.vi"("Host IP Address"="192.168.101.17") -> ("connected?"=w433:bool)  [unwired: 14 in]
    n224 = Scan Value(string=w454, format string="%f") -> (value=w445:dbl)  [unwired: 1 in, 1 out]
    n225 = Scan Value(string=w453, format string="%f") -> (value=w437:dbl)  [unwired: 1 in, 1 out]
    n226 = Not Equal?(x=w444, y=w445) -> (x != y?=w450:bool)
    n227 = Not Equal?(x=w435, y=w437) -> (x != y?=w442:bool)
    n228 = case shown="True" w450 {
      tunnel: w451 -> [w621 w630]
      tunnel: w449 -> [w622 w629]
      tunnel: [w622 w628] -> w448
      tunnel: w434 -> [_ w624]
      tunnel: w445 -> [_ w625]
      tunnel: [w621 w627] -> w447
      tunnel: [w620 w626] -> w446
      tunnel: w445 -> [_ w626]
      tunnel: w444 -> [w620 _]
      frame False {
      }
      frame True {
        n229 = Bundle(w624, w625) -> (w623:cluster{timestamp, dbl})  [unwired: 1 in]
        n230 = Replace Array Subset(array=w630, new element=w623, index=w629) -> (w627:cluster{"time stamp":timestamp, "Y":dbl}[])
        n231 = Increment(x=w629) -> (x+1=w628:i32)
      }
    }
    "CO Sensitivity" <- w447
    n232 = case shown="True" w442 {
      tunnel: w441 -> [w610 w619]
      tunnel: w440 -> [w611 w618]
      tunnel: [w611 w617] -> w438
      tunnel: w434 -> [_ w616]
      tunnel: w437 -> [_ w615]
      tunnel: [w610 w614] -> w439
      tunnel: [w609 w613] -> w436
      tunnel: w437 -> [_ w613]
      tunnel: w435 -> [w609 _]
      frame False {
      }
      frame True {
        n233 = Bundle(w616, w615) -> (w612:cluster{timestamp, dbl})  [unwired: 1 in]
        n234 = Replace Array Subset(array=w619, new element=w612, index=w618) -> (w614:cluster{"time stamp":timestamp, "Y":dbl}[])
        n235 = Increment(x=w618) -> (x+1=w617:i32)
      }
    }
    "CO Zero" <- w439
    n236 = case shown="False" w433 {
      tunnel: w432 -> [_ w608]
      tunnel: [FALSE w605] -> w431
      frame False {
      }
      frame True {
        n237 = Select(t=FALSE, s=w608, f=TRUE) -> (s? t:f=w605:bool)
      }
    }
    "Network to cRIO live status" <- w431
    n238 = Wait (ms)(milliseconds to wait=u32 1000) -> ()  [unwired: 1 out]
  }
  n239 = Obtain Queue(name (unnamed)="FGGA_Command", element data type=w55) -> (queue out=w2:refnum<queue>, error out=w1:errorcluster)  [unwired: 3 in, 1 out]
  n240 = while {
    tunnel: w2 -> [w632]
    tunnel: w1 -> [w631]
    tunnel: [w634] -> _
    tunnel: w13 -> [w633]
    stop <- FALSE stop-if-true
    # "FGGA UI Event Handler Loop"
    n241 = event shown="[5] \"Confirm Flight Number\": Value Change" {
      selector: _ -> [_ _ _ _ _ _ _ _ _ _ _ _ _ _ _ _ _]
      dyn-events: _ -> [_ _ _ _ _ _ _ _ _ _ _ _ _ _ _ _ _]
      timeout: _ -> [_ _ _ _ _ _ _ _ _ _ _ _ _ _ _ _ _]
      tunnel: w632 -> [w642 w646 w653 w660 w667 w674 w681 w688 w707 w816 w989 w1056 w1123 w1180 w1267 w1335 w1342]
      tunnel: w631 -> [w641 w645 w652 w659 w666 w673 w680 w687 w706 w815 w988 w1055 w1122 w1179 w1266 w1334 w1341]
      tunnel: [w636 w644 w651 w658 w665 w672 w679 w686 w693 w779 w981 w1048 w1115 w1166 w1253 w1333 w1340] -> w634
      tunnel: w633 -> [_ _ _ _ _ _ _ _ _ w803 _ _ _ _ _ _ _]
      event "V1": Value Change {
        n242 = event-data() -> ("NewVal"=w639:bool)  [unwired: 1 in]
        n243 = Bundle(cluster=T4 {"Message"="", "Message Data"=variant} ("Message Cluster"), "Message"="V1", "Message Data"=w639) -> (w637:T4)
        n244 = Enqueue Element(queue=w642, element=w637, error in (no error)=w641) -> (error out=w636:errorcluster)  [unwired: 1 in, 2 out]
      }
      event "V2": Value Change {
        n245 = event-data() -> ("NewVal"=w643:bool)  [unwired: 1 in]
        n246 = Bundle(cluster=T4 {"Message"="", "Message Data"=variant} ("Message Cluster"), "Message"="V2", "Message Data"=w643) -> (w647:T4)
        n247 = Enqueue Element(queue=w646, element=w647, error in (no error)=w645) -> (error out=w644:errorcluster)  [unwired: 1 in, 2 out]
      }
      event "V3": Value Change {
        n248 = event-data() -> ("NewVal"=w650:bool)  [unwired: 1 in]
        n249 = Bundle(cluster=T4 {"Message"="", "Message Data"=variant} ("Message Cluster"), "Message"="V3", "Message Data"=w650) -> (w654:T4)
        n250 = Enqueue Element(queue=w653, element=w654, error in (no error)=w652) -> (error out=w651:errorcluster)  [unwired: 1 in, 2 out]
      }
      event "V4": Value Change {
        n251 = event-data() -> ("NewVal"=w657:bool)  [unwired: 1 in]
        n252 = Bundle(cluster=T4 {"Message"="", "Message Data"=variant} ("Message Cluster"), "Message"="V4", "Message Data"=w657) -> (w661:T4)
        n253 = Enqueue Element(queue=w660, element=w661, error in (no error)=w659) -> (error out=w658:errorcluster)  [unwired: 1 in, 2 out]
      }
      event "FGGA Pump": Value Change {
        n254 = event-data() -> ("NewVal"=w664:bool)  [unwired: 1 in]
        n255 = Bundle(cluster=T4 {"Message"="", "Message Data"=variant} ("Message Cluster"), "Message"="FGGA_pump", "Message Data"=w664) -> (w668:T4)
        n256 = Enqueue Element(queue=w667, element=w668, error in (no error)=w666) -> (error out=w665:errorcluster)  [unwired: 1 in, 2 out]
      }
      event "Confirm Flight Number": Value Change {
        n257 = event-data() -> ()  [unwired: 1 in, 6 out]
        n258 = local read "Flight Number"() -> (w671:string)
        n259 = Bundle(cluster=T4 {"Message"="", "Message Data"=variant} ("Message Cluster"), "Message"="Flight Number", "Message Data"=w671) -> (w675:T4)
        n260 = Enqueue Element(queue=w674, element=w675, error in (no error)=w673) -> (error out=w672:errorcluster)  [unwired: 1 in, 2 out]
      }
      event "FGGA Restart": Value Change {
        n261 = event-data() -> ("NewVal"=w678:bool)  [unwired: 1 in]
        n262 = Bundle(cluster=T4 {"Message"="", "Message Data"=variant} ("Message Cluster"), "Message"="FGGA_restart", "Message Data"=w678) -> (w682:T4)
        n263 = Enqueue Element(queue=w681, element=w682, error in (no error)=w680) -> (error out=w679:errorcluster)  [unwired: 1 in, 2 out]
      }
      event "cRIO File IO Stop\n(USB Flash Drive Unmount)": Value Change {
        n264 = event-data() -> ("NewVal"=w685:bool)  [unwired: 1 in]
        n265 = Bundle(cluster=T4 {"Message"="", "Message Data"=variant} ("Message Cluster"), "Message"="Stop File Write", "Message Data"=w685) -> (w689:T4)
        n266 = Enqueue Element(queue=w688, element=w689, error in (no error)=w687) -> (error out=w686:errorcluster)  [unwired: 1 in, 2 out]
      }
      event "High Cal": Value Change {
        n267 = event-data() -> ()  [unwired: 1 in, 1 out]
        n268 = flat-sequence {
          tunnel: w707 -> [w712]
          tunnel: w706 -> [w711]
          tunnel: [w710] -> w705
          tunnel: [w709] -> w704
          tunnel: w705 -> [w728]
          tunnel: w704 -> [w727]
          tunnel: [w725] -> w702
          tunnel: [w724] -> w700
          tunnel: [w733] -> w703
          tunnel: w702 -> [w733]
          tunnel: [w732] -> w701
          tunnel: w700 -> [w732]
          tunnel: w703 -> [w743]
          tunnel: w701 -> [w742]
          tunnel: [w740] -> w698
          tunnel: [w739] -> w696
          tunnel: [w749] -> w699
          tunnel: w698 -> [w749]
          tunnel: [w748] -> w697
          tunnel: w696 -> [w748]
          tunnel: w699 -> [w759]
          tunnel: w697 -> [w758]
          tunnel: [w756] -> w695
          tunnel: [w755] -> w694
          tunnel: w695 -> [w773]
          tunnel: w694 -> [w772]
          tunnel: [w770] -> w692
          tunnel: [w778] -> w693
          tunnel: w692 -> [w778]
          frame #0 {
            w708 = TRUE
            n269 = Cluster To Array(cluster=T11 {"Message"="V2", "Message 2"="V3", "Message 3"="V4"}) -> (array=w713:string[])
            n270 = for {
              tunnel: w713 -> [w720] mode=indexing
              tunnel: w712 -> [w719]
              tunnel: w711 -> [w718]
              tunnel: [w717] -> w710
              tunnel: [w716] -> w709
              tunnel: w708 -> [w715]
              n271 = Bundle(cluster=T4 {"Message"="", "Message Data"=variant} ("Message Cluster"), "Message"=w720, "Message Data"=w715) -> (w722:T4)
              n272 = Enqueue Element(queue=w719, element=w722, error in (no error)=w718) -> (queue out=w717:refnum<queue>, error out=w716:errorcluster)  [unwired: 1 in, 1 out]
            }
            n273 = local write "V2"(w708) -> ()
            n274 = local write "V4"(w708) -> ()
            n275 = local write "V3"(w708) -> ()
          }
          frame #1 {
            n276 = local read "MFC_1 User Set Value"() -> (w723:dbl)
            n277 = local write "MFC_1\nSLPM Value"(w723) -> ()
            n278 = Bundle(cluster=T4 {"Message"="", "Message Data"=variant} ("Message Cluster"), "Message"="MFC_1", "Message Data"=w723) -> (w726:T4)
            n279 = Enqueue Element(queue=w728, element=w726, error in (no error)=w727) -> (queue out=w725:refnum<queue>, error out=w724:errorcluster)  [unwired: 1 in, 1 out]
          }
          frame #2 {
            n280 = for {
              N: 45 -> [w737]
              i -> [w736]
              n281 = Subtract(x=w737, y=w736) -> (x-y=w735:i32)
              n282 = Decrement(x=w735) -> (x-1=→"High Cal\nFlush Time Remain (sec)":i32)
              n283 = Wait (ms)(milliseconds to wait=u32 1000) -> ()  [unwired: 1 out]
            }
          }
          frame #3 {
            w741 = TRUE
            n284 = Bundle(cluster=T4 {"Message"="", "Message Data"=variant} ("Message Cluster"), "Message"="V1", "Message Data"=w741) -> (w744:T4)
            n285 = local write "V1"(w741) -> ()
            n286 = Enqueue Element(queue=w743, element=w744, error in (no error)=w742) -> (queue out=w740:refnum<queue>, error out=w739:errorcluster)  [unwired: 1 in, 1 out]
          }
          frame #4 {
            n287 = for {
              N: 60 -> [w753]
              i -> [w752]
              n288 = Subtract(x=w753, y=w752) -> (x-y=w751:i32)
              n289 = Decrement(x=w751) -> (x-1=→"High Cal\nCal Time Remain (sec)":i32)
              n290 = Wait (ms)(milliseconds to wait=u32 1000) -> ()  [unwired: 1 out]
            }
          }
          frame #5 {
            w757 = FALSE
            n291 = Cluster To Array(cluster=T12 {"Message"="V2", "Message 2"="V3", "Message 3"="V4", "Message 4"="V1"}) -> (array=w760:string[])
            n292 = for {
              tunnel: w760 -> [w767] mode=indexing
              tunnel: [w766] -> w756
              tunnel: [w765] -> w755
              tunnel: w757 -> [w764]
              tunnel: w759 -> [w763]
              tunnel: w758 -> [w762]
              n293 = Bundle(cluster=T4 {"Message"="", "Message Data"=variant} ("Message Cluster"), "Message"=w767, "Message Data"=w764) -> (w769:T4)
              n294 = Enqueue Element(queue=w763, element=w769, error in (no error)=w762) -> (queue out=w766:refnum<queue>, error out=w765:errorcluster)  [unwired: 1 in, 1 out]
            }
            n295 = local write "V2"(w757) -> ()
            n296 = local write "V4"(w757) -> ()
            n297 = local write "V3"(w757) -> ()
            n298 = local write "V1"(w757) -> ()
          }
          frame #6 {
            w771 = 0.0 ("MFC_1\nSLPM Value")
            n299 = local write "MFC_1\nSLPM Value"(w771) -> ()
            n300 = Bundle(cluster=T4 {"Message"="", "Message Data"=variant} ("Message Cluster"), "Message"="MFC_1", "Message Data"=w771) -> (w775:T4)
            n301 = Enqueue Element(queue=w773, element=w775, error in (no error)=w772) -> (error out=w770:errorcluster)  [unwired: 1 in, 2 out]
          }
          frame #7 {
            n302 = local write "High Cal"(FALSE ("High Cal")) -> ()
          }
        }
      }
      event "Span Cal": Value Change {
        n303 = event-data() -> ()  [unwired: 1 in, 1 out]
        n304 = flat-sequence {
          tunnel: w816 -> [w822]
          tunnel: w815 -> [w821]
          tunnel: [w820] -> w814
          tunnel: [w819] -> w813
          tunnel: w814 -> [w838]
          tunnel: w813 -> [w837]
          tunnel: [w835] -> w811
          tunnel: [w834] -> w809
          tunnel: [w843] -> w812
          tunnel: w811 -> [w843]
          tunnel: [w842] -> w810
          tunnel: w809 -> [w842]
          tunnel: w812 -> [w849]
          tunnel: w810 -> [w850]
          tunnel: [w850] -> w785
          tunnel: w803 -> [w851]
          tunnel: [w851] -> w783
          tunnel: [w849] -> w781
          tunnel: w785 -> [w859]
          tunnel: [w859] -> w784
          tunnel: w783 -> [w858]
          tunnel: [w858] -> w782
          tunnel: w781 -> [w856]
          tunnel: [w856] -> w780
          tunnel: [w860] -> w802
          tunnel: w784 -> [w863]
          tunnel: [w862] -> w801
          tunnel: w782 -> [w872]
          tunnel: w780 -> [w861]
          tunnel: [w875] -> w808
          tunnel: w802 -> [w875]
          tunnel: [w874] -> w807
          tunnel: w801 -> [w874]
          tunnel: w808 -> [w885]
          tunnel: w807 -> [w884]
          tunnel: [w882] -> w806
          tunnel: [w881] -> w805
          tunnel: w806 -> [w900]
          tunnel: w805 -> [w899]
          tunnel: [w897] -> w804
          tunnel: [w896] -> w798
          tunnel: w804 -> [w906]
          tunnel: [w906] -> w800
          tunnel: [w904] -> w799
          tunnel: w798 -> [w904]
          tunnel: w800 -> [w911]
          tunnel: w799 -> [w913]
          tunnel: [w910] -> w797
          tunnel: [w907] -> w796
          tunnel: w797 -> [w927]
          tunnel: w796 -> [w925]
          tunnel: [w924] -> w795
          tunnel: [w923] -> w792
          tunnel: w795 -> [w932]
          tunnel: [w932] -> w794
          tunnel: [w931] -> w793
          tunnel: w792 -> [w931]
          tunnel: w794 -> [w944]
          tunnel: w793 -> [w942]
          tunnel: [w940] -> w790
          tunnel: [w939] -> w788
          tunnel: [w948] -> w791
          tunnel: w790 -> [w948]
          tunnel: [w947] -> w789
          tunnel: w788 -> [w947]
          tunnel: w791 -> [w959]
          tunnel: w789 -> [w958]
          tunnel: [w956] -> w787
          tunnel: [w955] -> w786
          tunnel: w787 -> [w974]
          tunnel: w786 -> [w973]
          tunnel: [w970] -> w779
          frame #0 {
            w818 = TRUE
            n305 = Cluster To Array(cluster=T11 {"Message"="V2", "Message 2"="V3", "Message 3"="V4"}) -> (array=w823:string[])
            n306 = for {
              tunnel: w823 -> [w830] mode=indexing
              tunnel: w822 -> [w829]
              tunnel: w821 -> [w828]
              tunnel: [w827] -> w820
              tunnel: [w826] -> w819
              tunnel: w818 -> [w825]
              n307 = Bundle(cluster=T4 {"Message"="", "Message Data"=variant} ("Message Cluster"), "Message"=w830, "Message Data"=w825) -> (w832:T4)
              n308 = Enqueue Element(queue=w829, element=w832, error in (no error)=w828) -> (queue out=w827:refnum<queue>, error out=w826:errorcluster)  [unwired: 1 in, 1 out]
            }
            n309 = local write "High Cal"(TRUE ("High Cal")) -> ()
            n310 = local write "V2"(w818) -> ()
            n311 = local write "V4"(w818) -> ()
            n312 = local write "V3"(w818) -> ()
          }
          frame #1 {
            n313 = local read "MFC_1 User Set Value"() -> (w833:dbl)
            n314 = local write "MFC_1\nSLPM Value"(w833) -> ()
            n315 = Bundle(cluster=T4 {"Message"="", "Message Data"=variant} ("Message Cluster"), "Message"="MFC_1", "Message Data"=w833) -> (w836:T4)
            n316 = Enqueue Element(queue=w838, element=w836, error in (no error)=w837) -> (queue out=w835:refnum<queue>, error out=w834:errorcluster)  [unwired: 1 in, 1 out]
          }
          frame #2 {
            n317 = for {
              N: 45 -> [w847]
              i -> [w846]
              n318 = Subtract(x=w847, y=w846) -> (x-y=w845:i32)
              n319 = Decrement(x=w845) -> (x-1=w844:i32)
              n320 = local write "High Cal\nFlush Time Remain (sec)"(w844) -> ()
              n321 = Wait (ms)(milliseconds to wait=u32 1000) -> ()  [unwired: 1 out]
            }
          }
          frame #3 {
            n322 = Bundle(cluster=T4 {"Message"="", "Message Data"=variant} ("Message Cluster"), "Message"="CO CAL", "Message Data"=TRUE) -> (w853:T4)
            n323 = Enqueue Element(queue=w851, element=w853) -> ()  [unwired: 2 in, 3 out]
          }
          frame #4 {
            # "To Ensure\nCO CAL\nis certain"
            n324 = Wait (ms)(milliseconds to wait=u32 1000) -> ()  [unwired: 1 out]
          }
          frame #5 {
            w867 = TRUE
            n325 = Bundle(cluster=T4 {"Message"="", "Message Data"=variant} ("Message Cluster"), "Message"="CO CAL", "Message Data"=FALSE) -> (w868:T4)
            n326 = Bundle(cluster=T4 {"Message"="", "Message Data"=variant} ("Message Cluster"), "Message"="V1", "Message Data"=w867) -> (w866:T4)
            n327 = local write "V1"(w867) -> ()
            n328 = Enqueue Element(queue=w872, element=w868) -> ()  [unwired: 2 in, 3 out]
            n329 = Enqueue Element(queue=w861, element=w866, error in (no error)=w863) -> (queue out=w860:refnum<queue>, error out=w862:errorcluster)  [unwired: 1 in, 1 out]
          }
          frame #6 {
            n330 = for {
              N: 60 -> [w879]
              i -> [w878]
              n331 = Subtract(x=w879, y=w878) -> (x-y=w877:i32)
              n332 = Decrement(x=w877) -> (x-1=w876:i32)
              n333 = local write "High Cal\nCal Time Remain (sec)"(w876) -> ()
              n334 = Wait (ms)(milliseconds to wait=u32 1000) -> ()  [unwired: 1 out]
            }
          }
          frame #7 {
            w883 = FALSE
            n335 = Cluster To Array(cluster=T12 {"Message"="V2", "Message 2"="V3", "Message 3"="V4", "Message 4"="V1"}) -> (array=w886:string[])
            n336 = for {
              tunnel: w886 -> [w893] mode=indexing
              tunnel: [w892] -> w882
              tunnel: [w891] -> w881
              tunnel: w883 -> [w890]
              tunnel: w885 -> [w889]
              tunnel: w884 -> [w888]
              n337 = Bundle(cluster=T4 {"Message"="", "Message Data"=variant} ("Message Cluster"), "Message"=w893, "Message Data"=w890) -> (w895:T4)
              n338 = Enqueue Element(queue=w889, element=w895, error in (no error)=w888) -> (queue out=w892:refnum<queue>, error out=w891:errorcluster)  [unwired: 1 in, 1 out]
            }
            n339 = local write "V2"(w883) -> ()
            n340 = local write "V4"(w883) -> ()
            n341 = local write "V3"(w883) -> ()
            n342 = local write "V1"(w883) -> ()
          }
          frame #8 {
            w898 = 0.0 ("MFC_1\nSLPM Value")
            n343 = local write "MFC_1\nSLPM Value"(w898) -> ()
            n344 = Bundle(cluster=T4 {"Message"="", "Message Data"=variant} ("Message Cluster"), "Message"="MFC_1", "Message Data"=w898) -> (w902:T4)
            n345 = Enqueue Element(queue=w900, element=w902, error in (no error)=w899) -> (queue out=w896:refnum<queue>, error out=w897:errorcluster)  [unwired: 1 in, 1 out]
          }
          frame #9 {
            n346 = local write "High Cal"(FALSE ("High Cal")) -> ()
          }
          frame #10 {
            w908 = TRUE
            n347 = Cluster To Array(cluster=cluster{"Message":string, "Message 3":string} {"Message"="V2", "Message 3"="V4"}) -> (array=w914:string[])
            n348 = for {
              tunnel: w914 -> [w920] mode=indexing
              tunnel: w913 -> [w919]
              tunnel: [w918] -> w907
              tunnel: [w917] -> w910
              tunnel: w908 -> [w916]
              tunnel: w911 -> [w915]
              n349 = Bundle(cluster=T4 {"Message"="", "Message Data"=variant} ("Message Cluster"), "Message"=w920, "Message Data"=w916) -> (w922:T4)
              n350 = Enqueue Element(queue=w919, element=w922, error in (no error)=w915) -> (queue out=w918:refnum<queue>, error out=w917:errorcluster)  [unwired: 1 in, 1 out]
            }
            n351 = local write "V4"(w908) -> ()
            n352 = local write "V2"(w908) -> ()
            n353 = local write "Low Cal"(TRUE ("Low Cal")) -> ()
          }
          frame #11 {
            n354 = local read "MFC_1 User Set Value"() -> (w928:dbl)
            n355 = local write "MFC_1\nSLPM Value"(w928) -> ()
            n356 = Bundle(cluster=T4 {"Message"="", "Message Data"=variant} ("Message Cluster"), "Message"="MFC_1", "Message Data"=w928) -> (w929:T4)
            n357 = Enqueue Element(queue=w925, element=w929, error in (no error)=w927) -> (queue out=w924:refnum<queue>, error out=w923:errorcluster)  [unwired: 1 in, 1 out]
          }
          frame #12 {
            n358 = for {
              N: 45 -> [w937]
              i -> [w936]
              n359 = Subtract(x=w937, y=w936) -> (x-y=w935:i32)
              n360 = Decrement(x=w935) -> (x-1=w934:i32)
              n361 = local write "Low Cal\nFlush Time Remain (sec)"(w934) -> ()
              n362 = Wait (ms)(milliseconds to wait=u32 1000) -> ()  [unwired: 1 out]
            }
          }
          frame #13 {
            w941 = TRUE
            n363 = local write "V1"(w941) -> ()
            n364 = Bundle(cluster=T4 {"Message"="", "Message Data"=variant} ("Message Cluster"), "Message"="V1", "Message Data"=w941) -> (w945:T4)
            n365 = Enqueue Element(queue=w944, element=w945, error in (no error)=w942) -> (queue out=w940:refnum<queue>, error out=w939:errorcluster)  [unwired: 1 in, 1 out]
          }
          frame #14 {
            n366 = for {
              N: 60 -> [w953]
              i -> [w952]
              n367 = Subtract(x=w953, y=w952) -> (x-y=w951:i32)
              n368 = Decrement(x=w951) -> (x-1=w950:i32)
              n369 = local write "Low Cal\nCal Time Remain (sec)"(w950) -> ()
              n370 = Wait (ms)(milliseconds to wait=u32 1000) -> ()  [unwired: 1 out]
            }
          }
          frame #15 {
            w957 = FALSE
            n371 = Cluster To Array(cluster=T13 {"Message"="V2", "Message 3"="V4", "Message 4"="V1"}) -> (array=w960:string[])
            n372 = for {
              tunnel: w960 -> [w967] mode=indexing
              tunnel: [w966] -> w956
              tunnel: [w965] -> w955
              tunnel: w957 -> [w964]
              tunnel: w959 -> [w963]
              tunnel: w958 -> [w962]
              n373 = Bundle(cluster=T4 {"Message"="", "Message Data"=variant} ("Message Cluster"), "Message"=w967, "Message Data"=w964) -> (w969:T4)
              n374 = Enqueue Element(queue=w963, element=w969, error in (no error)=w962) -> (queue out=w966:refnum<queue>, error out=w965:errorcluster)  [unwired: 1 in, 1 out]
            }
            n375 = local write "V1"(w957) -> ()
            n376 = local write "V2"(w957) -> ()
            n377 = local write "V4"(w957) -> ()
          }
          frame #16 {
            w971 = FALSE
            w972 = 0.0 ("MFC_1\nSLPM Value")
            n378 = local write "MFC_1\nSLPM Value"(w972) -> ()
            n379 = local write "Span Cal"(w971) -> ()
            n380 = local write "Low Cal"(w971) -> ()
            n381 = Bundle(cluster=T4 {"Message"="", "Message Data"=variant} ("Message Cluster"), "Message"="MFC_1", "Message Data"=w972) -> (w976:T4)
            n382 = Enqueue Element(queue=w974, element=w976, error in (no error)=w973) -> (error out=w970:errorcluster)  [unwired: 1 in, 2 out]
          }
        }
      }
      event "Flush High Tank": Value Change {
        n383 = event-data() -> ()  [unwired: 1 in, 1 out]
        n384 = flat-sequence {
          tunnel: w989 -> [w994]
          tunnel: w988 -> [w993]
          tunnel: [w992] -> w987
          tunnel: [w991] -> w986
          tunnel: w987 -> [w1010]
          tunnel: w986 -> [w1009]
          tunnel: [w1007] -> w985
          tunnel: [w1006] -> w984
          tunnel: w985 -> [w1013]
          tunnel: w984 -> [w1014]
          tunnel: [w1014] -> w979
          tunnel: [w1013] -> w978
          tunnel: [w1024] -> w983
          tunnel: [w1023] -> w982
          tunnel: w979 -> [w1022]
          tunnel: w978 -> [w1021]
          tunnel: w983 -> [w1039]
          tunnel: w982 -> [w1038]
          tunnel: [w1036] -> w980
          tunnel: [w1044] -> w981
          tunnel: w980 -> [w1044]
          frame #0 {
            w990 = TRUE
            n385 = Cluster To Array(cluster=T11 {"Message"="V2", "Message 2"="V3", "Message 3"="V4"}) -> (array=w995:string[])
            n386 = for {
              tunnel: w995 -> [w1002] mode=indexing
              tunnel: w994 -> [w1001]
              tunnel: w993 -> [w1000]
              tunnel: [w999] -> w992
              tunnel: [w998] -> w991
              tunnel: w990 -> [w997]
              n387 = Bundle(cluster=T4 {"Message"="", "Message Data"=variant} ("Message Cluster"), "Message"=w1002, "Message Data"=w997) -> (w1004:T4)
              n388 = Enqueue Element(queue=w1001, element=w1004, error in (no error)=w1000) -> (queue out=w999:refnum<queue>, error out=w998:errorcluster)  [unwired: 1 in, 1 out]
            }
            n389 = local write "V2"(w990) -> ()
            n390 = local write "V4"(w990) -> ()
            n391 = local write "V3"(w990) -> ()
          }
          frame #1 {
            n392 = local read "MFC_1 User Set Value"() -> (w1005:dbl)
            n393 = local write "MFC_1\nSLPM Value"(w1005) -> ()
            n394 = Bundle(cluster=T4 {"Message"="", "Message Data"=variant} ("Message Cluster"), "Message"="MFC_1", "Message Data"=w1005) -> (w1008:T4)
            n395 = Enqueue Element(queue=w1010, element=w1008, error in (no error)=w1009) -> (queue out=w1007:refnum<queue>, error out=w1006:errorcluster)  [unwired: 1 in, 1 out]
          }
          frame #2 {
            n396 = for {
              N: 15 -> [w1019]
              i -> [w1018]
              n397 = Subtract(x=w1019, y=w1018) -> (x-y=w1017:i32)
              n398 = Decrement(x=w1017) -> (x-1=→"Flush High Tank\nTime Remain (sec)":i32)
              n399 = Wait (ms)(milliseconds to wait=u32 1000) -> ()  [unwired: 1 out]
            }
          }
          frame #3 {
            w1025 = FALSE
            n400 = Cluster To Array(cluster=T11 {"Message"="V2", "Message 2"="V3", "Message 3"="V4"}) -> (array=w1026:string[])
            n401 = for {
              tunnel: w1026 -> [w1033] mode=indexing
              tunnel: [w1032] -> w1024
              tunnel: [w1031] -> w1023
              tunnel: w1025 -> [w1030]
              tunnel: w1021 -> [w1029]
              tunnel: w1022 -> [w1028]
              n402 = Bundle(cluster=T4 {"Message"="", "Message Data"=variant} ("Message Cluster"), "Message"=w1033, "Message Data"=w1030) -> (w1035:T4)
              n403 = Enqueue Element(queue=w1029, element=w1035, error in (no error)=w1028) -> (queue out=w1032:refnum<queue>, error out=w1031:errorcluster)  [unwired: 1 in, 1 out]
            }
            n404 = local write "V2"(w1025) -> ()
            n405 = local write "V4"(w1025) -> ()
            n406 = local write "V3"(w1025) -> ()
          }
          frame #4 {
            w1037 = 0.0 ("MFC_1\nSLPM Value")
            n407 = local write "MFC_1\nSLPM Value"(w1037) -> ()
            n408 = Bundle(cluster=T4 {"Message"="", "Message Data"=variant} ("Message Cluster"), "Message"="MFC_1", "Message Data"=w1037) -> (w1041:T4)
            n409 = Enqueue Element(queue=w1039, element=w1041, error in (no error)=w1038) -> (error out=w1036:errorcluster)  [unwired: 1 in, 2 out]
          }
          frame #5 {
            n410 = local write "Flush High Tank"(FALSE ("High Cal")) -> ()
          }
        }
      }
      event "Flush Low Tank": Value Change {
        n411 = event-data() -> ()  [unwired: 1 in, 1 out]
        n412 = flat-sequence {
          tunnel: w1056 -> [w1061]
          tunnel: w1055 -> [w1060]
          tunnel: [w1059] -> w1054
          tunnel: [w1058] -> w1053
          tunnel: w1054 -> [w1077]
          tunnel: w1053 -> [w1076]
          tunnel: [w1074] -> w1052
          tunnel: [w1073] -> w1051
          tunnel: w1052 -> [w1080]
          tunnel: w1051 -> [w1081]
          tunnel: [w1081] -> w1046
          tunnel: [w1080] -> w1045
          tunnel: [w1091] -> w1050
          tunnel: [w1090] -> w1049
          tunnel: w1046 -> [w1089]
          tunnel: w1045 -> [w1088]
          tunnel: w1050 -> [w1106]
          tunnel: w1049 -> [w1105]
          tunnel: [w1103] -> w1047
          tunnel: [w1111] -> w1048
          tunnel: w1047 -> [w1111]
          frame #0 {
            w1057 = TRUE
            n413 = Cluster To Array(cluster=cluster{"Message":string, "Message 3":string} {"Message"="V2", "Message 3"="V4"}) -> (array=w1062:string[])
            n414 = for {
              tunnel: w1062 -> [w1069] mode=indexing
              tunnel: w1061 -> [w1068]
              tunnel: w1060 -> [w1067]
              tunnel: [w1066] -> w1059
              tunnel: [w1065] -> w1058
              tunnel: w1057 -> [w1064]
              n415 = Bundle(cluster=T4 {"Message"="", "Message Data"=variant} ("Message Cluster"), "Message"=w1069, "Message Data"=w1064) -> (w1071:T4)
              n416 = Enqueue Element(queue=w1068, element=w1071, error in (no error)=w1067) -> (queue out=w1066:refnum<queue>, error out=w1065:errorcluster)  [unwired: 1 in, 1 out]
            }
            n417 = local write "V2"(w1057) -> ()
            n418 = local write "V4"(w1057) -> ()
          }
          frame #1 {
            n419 = local read "MFC_1 User Set Value"() -> (w1072:dbl)
            n420 = local write "MFC_1\nSLPM Value"(w1072) -> ()
            n421 = Bundle(cluster=T4 {"Message"="", "Message Data"=variant} ("Message Cluster"), "Message"="MFC_1", "Message Data"=w1072) -> (w1075:T4)
            n422 = Enqueue Element(queue=w1077, element=w1075, error in (no error)=w1076) -> (queue out=w1074:refnum<queue>, error out=w1073:errorcluster)  [unwired: 1 in, 1 out]
          }
          frame #2 {
            n423 = for {
              N: 15 -> [w1086]
              i -> [w1085]
              n424 = Subtract(x=w1086, y=w1085) -> (x-y=w1084:i32)
              n425 = Decrement(x=w1084) -> (x-1=→"Flush Low Tank\nTime Remain (sec)":i32)
              n426 = Wait (ms)(milliseconds to wait=u32 1000) -> ()  [unwired: 1 out]
            }
          }
          frame #3 {
            w1092 = FALSE
            n427 = Cluster To Array(cluster=cluster{"Message":string, "Message 3":string} {"Message"="V2", "Message 3"="V4"}) -> (array=w1093:string[])
            n428 = for {
              tunnel: w1093 -> [w1100] mode=indexing
              tunnel: [w1099] -> w1091
              tunnel: [w1098] -> w1090
              tunnel: w1092 -> [w1097]
              tunnel: w1088 -> [w1096]
              tunnel: w1089 -> [w1095]
              n429 = Bundle(cluster=T4 {"Message"="", "Message Data"=variant} ("Message Cluster"), "Message"=w1100, "Message Data"=w1097) -> (w1102:T4)
              n430 = Enqueue Element(queue=w1096, element=w1102, error in (no error)=w1095) -> (queue out=w1099:refnum<queue>, error out=w1098:errorcluster)  [unwired: 1 in, 1 out]
            }
            n431 = local write "V2"(w1092) -> ()
            n432 = local write "V4"(w1092) -> ()
          }
          frame #4 {
            w1104 = 0.0 ("MFC_1\nSLPM Value")
            n433 = local write "MFC_1\nSLPM Value"(w1104) -> ()
            n434 = Bundle(cluster=T4 {"Message"="", "Message Data"=variant} ("Message Cluster"), "Message"="MFC_1", "Message Data"=w1104) -> (w1108:T4)
            n435 = Enqueue Element(queue=w1106, element=w1108, error in (no error)=w1105) -> (error out=w1103:errorcluster)  [unwired: 1 in, 2 out]
          }
          frame #5 {
            n436 = local write "Flush Low Tank"(FALSE ("High Cal")) -> ()
          }
        }
      }
      event "Flush Target Tank": Value Change {
        n437 = event-data() -> ()  [unwired: 1 in, 1 out]
        n438 = flat-sequence {
          tunnel: w1123 -> [w1131]
          tunnel: w1122 -> [w1130]
          tunnel: [w1129] -> w1121
          tunnel: [w1128] -> w1120
          tunnel: w1121 -> [w1137]
          tunnel: w1120 -> [w1136]
          tunnel: [w1134] -> w1119
          tunnel: [w1133] -> w1118
          tunnel: w1119 -> [w1140]
          tunnel: w1118 -> [w1141]
          tunnel: [w1141] -> w1113
          tunnel: [w1140] -> w1112
          tunnel: [w1154] -> w1117
          tunnel: [w1153] -> w1116
          tunnel: w1113 -> [w1152]
          tunnel: w1112 -> [w1151]
          tunnel: w1117 -> [w1159]
          tunnel: w1116 -> [w1158]
          tunnel: [w1156] -> w1114
          tunnel: [w1164] -> w1115
          tunnel: w1114 -> [w1164]
          frame #0 {
            w1127 = TRUE
            n439 = local write "V4"(w1127) -> ()
            n440 = Bundle(cluster=T4 {"Message"="", "Message Data"=variant} ("Message Cluster"), "Message"="V4" ("Message 3"), "Message Data"=w1127) -> (w1126:T4)
            n441 = Enqueue Element(queue=w1131, element=w1126, error in (no error)=w1130) -> (queue out=w1129:refnum<queue>, error out=w1128:errorcluster)  [unwired: 1 in, 1 out]
          }
          frame #1 {
            n442 = local read "MFC_1 User Set Value"() -> (w1132:dbl)
            n443 = local write "MFC_1\nSLPM Value"(w1132) -> ()
            n444 = Bundle(cluster=T4 {"Message"="", "Message Data"=variant} ("Message Cluster"), "Message"="MFC_1", "Message Data"=w1132) -> (w1135:T4)
            n445 = Enqueue Element(queue=w1137, element=w1135, error in (no error)=w1136) -> (queue out=w1134:refnum<queue>, error out=w1133:errorcluster)  [unwired: 1 in, 1 out]
          }
          frame #2 {
            n446 = for {
              N: 15 -> [w1146]
              i -> [w1145]
              n447 = Subtract(x=w1146, y=w1145) -> (x-y=w1144:i32)
              n448 = Decrement(x=w1144) -> (x-1=→"Flush Target Tank\nTime Remain (sec)":i32)
              n449 = Wait (ms)(milliseconds to wait=u32 1000) -> ()  [unwired: 1 out]
            }
          }
          frame #3 {
            w1155 = FALSE
            n450 = Bundle(cluster=T4 {"Message"="", "Message Data"=variant} ("Message Cluster"), "Message"="V4" ("Message 3"), "Message Data"=w1155) -> (w1150:T4)
            n451 = local write "V4"(w1155) -> ()
            n452 = Enqueue Element(queue=w1151, element=w1150, error in (no error)=w1152) -> (queue out=w1154:refnum<queue>, error out=w1153:errorcluster)  [unwired: 1 in, 1 out]
          }
          frame #4 {
            w1157 = 0.0 ("MFC_1\nSLPM Value")
            n453 = local write "MFC_1\nSLPM Value"(w1157) -> ()
            n454 = Bundle(cluster=T4 {"Message"="", "Message Data"=variant} ("Message Cluster"), "Message"="MFC_1", "Message Data"=w1157) -> (w1161:T4)
            n455 = Enqueue Element(queue=w1159, element=w1161, error in (no error)=w1158) -> (error out=w1156:errorcluster)  [unwired: 1 in, 2 out]
          }
          frame #5 {
            n456 = local write "Flush Target Tank"(FALSE ("High Cal")) -> ()
          }
        }
      }
      event "Low Cal": Value Change {
        n457 = event-data() -> ()  [unwired: 1 in, 1 out]
        n458 = flat-sequence {
          tunnel: w1180 -> [w1185]
          tunnel: w1179 -> [w1184]
          tunnel: [w1183] -> w1178
          tunnel: [w1182] -> w1177
          tunnel: w1178 -> [w1201]
          tunnel: w1177 -> [w1200]
          tunnel: [w1198] -> w1175
          tunnel: [w1197] -> w1173
          tunnel: [w1206] -> w1176
          tunnel: w1175 -> [w1206]
          tunnel: [w1205] -> w1174
          tunnel: w1173 -> [w1205]
          tunnel: w1176 -> [w1216]
          tunnel: w1174 -> [w1215]
          tunnel: [w1213] -> w1171
          tunnel: [w1212] -> w1169
          tunnel: [w1222] -> w1172
          tunnel: w1171 -> [w1222]
          tunnel: [w1221] -> w1170
          tunnel: w1169 -> [w1221]
          tunnel: w1172 -> [w1232]
          tunnel: w1170 -> [w1231]
          tunnel: [w1229] -> w1168
          tunnel: [w1228] -> w1167
          tunnel: w1168 -> [w1246]
          tunnel: w1167 -> [w1245]
          tunnel: [w1243] -> w1165
          tunnel: [w1251] -> w1166
          tunnel: w1165 -> [w1251]
          frame #0 {
            w1181 = TRUE
            n459 = Cluster To Array(cluster=cluster{"Message":string, "Message 3":string} {"Message"="V2", "Message 3"="V4"}) -> (array=w1186:string[])
            n460 = for {
              tunnel: w1186 -> [w1193] mode=indexing
              tunnel: w1185 -> [w1192]
              tunnel: w1184 -> [w1191]
              tunnel: [w1190] -> w1183
              tunnel: [w1189] -> w1182
              tunnel: w1181 -> [w1188]
              n461 = Bundle(cluster=T4 {"Message"="", "Message Data"=variant} ("Message Cluster"), "Message"=w1193, "Message Data"=w1188) -> (w1195:T4)
              n462 = Enqueue Element(queue=w1192, element=w1195, error in (no error)=w1191) -> (queue out=w1190:refnum<queue>, error out=w1189:errorcluster)  [unwired: 1 in, 1 out]
            }
            n463 = local write "V2"(w1181) -> ()
            n464 = local write "V4"(w1181) -> ()
          }
          frame #1 {
            n465 = local read "MFC_1 User Set Value"() -> (w1196:dbl)
            n466 = local write "MFC_1\nSLPM Value"(w1196) -> ()
            n467 = Bundle(cluster=T4 {"Message"="", "Message Data"=variant} ("Message Cluster"), "Message"="MFC_1", "Message Data"=w1196) -> (w1199:T4)
            n468 = Enqueue Element(queue=w1201, element=w1199, error in (no error)=w1200) -> (queue out=w1198:refnum<queue>, error out=w1197:errorcluster)  [unwired: 1 in, 1 out]
          }
          frame #2 {
            n469 = for {
              N: 45 -> [w1210]
              i -> [w1209]
              n470 = Subtract(x=w1210, y=w1209) -> (x-y=w1208:i32)
              n471 = Decrement(x=w1208) -> (x-1=→"Low Cal\nFlush Time Remain (sec)":i32)
              n472 = Wait (ms)(milliseconds to wait=u32 1000) -> ()  [unwired: 1 out]
            }
          }
          frame #3 {
            w1214 = TRUE
            n473 = Bundle(cluster=T4 {"Message"="", "Message Data"=variant} ("Message Cluster"), "Message"="V1", "Message Data"=w1214) -> (w1217:T4)
            n474 = local write "V1"(w1214) -> ()
            n475 = Enqueue Element(queue=w1216, element=w1217, error in (no error)=w1215) -> (queue out=w1213:refnum<queue>, error out=w1212:errorcluster)  [unwired: 1 in, 1 out]
          }
          frame #4 {
            n476 = for {
              N: 60 -> [w1226]
              i -> [w1225]
              n477 = Subtract(x=w1226, y=w1225) -> (x-y=w1224:i32)
              n478 = Decrement(x=w1224) -> (x-1=→"Low Cal\nCal Time Remain (sec)":i32)
              n479 = Wait (ms)(milliseconds to wait=u32 1000) -> ()  [unwired: 1 out]
            }
          }
          frame #5 {
            w1230 = FALSE
            n480 = Cluster To Array(cluster=T13 {"Message"="V2", "Message 3"="V4", "Message 4"="V1"}) -> (array=w1233:string[])
            n481 = for {
              tunnel: w1233 -> [w1240] mode=indexing
              tunnel: [w1239] -> w1229
              tunnel: [w1238] -> w1228
              tunnel: w1230 -> [w1237]
              tunnel: w1232 -> [w1236]
              tunnel: w1231 -> [w1235]
              n482 = Bundle(cluster=T4 {"Message"="", "Message Data"=variant} ("Message Cluster"), "Message"=w1240, "Message Data"=w1237) -> (w1242:T4)
              n483 = Enqueue Element(queue=w1236, element=w1242, error in (no error)=w1235) -> (queue out=w1239:refnum<queue>, error out=w1238:errorcluster)  [unwired: 1 in, 1 out]
            }
            n484 = local write "V2"(w1230) -> ()
            n485 = local write "V4"(w1230) -> ()
            n486 = local write "V1"(w1230) -> ()
          }
          frame #6 {
            w1244 = 0.0 ("MFC_1\nSLPM Value")
            n487 = local write "MFC_1\nSLPM Value"(w1244) -> ()
            n488 = Bundle(cluster=T4 {"Message"="", "Message Data"=variant} ("Message Cluster"), "Message"="MFC_1", "Message Data"=w1244) -> (w1248:T4)
            n489 = Enqueue Element(queue=w1246, element=w1248, error in (no error)=w1245) -> (error out=w1243:errorcluster)  [unwired: 1 in, 2 out]
          }
          frame #7 {
            n490 = local write "Low Cal"(FALSE ("High Cal")) -> ()
          }
        }
      }
      event "Target Cal": Value Change {
        n491 = event-data() -> ()  [unwired: 1 in, 1 out]
        n492 = flat-sequence {
          tunnel: w1267 -> [w1275]
          tunnel: w1266 -> [w1274]
          tunnel: [w1273] -> w1265
          tunnel: [w1272] -> w1264
          tunnel: w1265 -> [w1281]
          tunnel: w1264 -> [w1280]
          tunnel: [w1278] -> w1262
          tunnel: [w1277] -> w1260
          tunnel: [w1286] -> w1263
          tunnel: w1262 -> [w1286]
          tunnel: [w1285] -> w1261
          tunnel: w1260 -> [w1285]
          tunnel: w1263 -> [w1296]
          tunnel: w1261 -> [w1295]
          tunnel: [w1293] -> w1258
          tunnel: [w1292] -> w1256
          tunnel: [w1302] -> w1259
          tunnel: w1258 -> [w1302]
          tunnel: [w1301] -> w1257
          tunnel: w1256 -> [w1301]
          tunnel: w1259 -> [w1311]
          tunnel: w1257 -> [w1310]
          tunnel: [w1308] -> w1255
          tunnel: [w1309] -> w1254
          tunnel: w1255 -> [w1326]
          tunnel: w1254 -> [w1325]
          tunnel: [w1323] -> w1252
          tunnel: [w1331] -> w1253
          tunnel: w1252 -> [w1331]
          frame #0 {
            w1271 = TRUE
            n493 = local write "V4"(w1271) -> ()
            n494 = Bundle(cluster=T4 {"Message"="", "Message Data"=variant} ("Message Cluster"), "Message"="V4" ("Message 3"), "Message Data"=w1271) -> (w1270:T4)
            n495 = Enqueue Element(queue=w1275, element=w1270, error in (no error)=w1274) -> (queue out=w1273:refnum<queue>, error out=w1272:errorcluster)  [unwired: 1 in, 1 out]
          }
          frame #1 {
            n496 = local read "MFC_1 User Set Value"() -> (w1276:dbl)
            n497 = local write "MFC_1\nSLPM Value"(w1276) -> ()
            n498 = Bundle(cluster=T4 {"Message"="", "Message Data"=variant} ("Message Cluster"), "Message"="MFC_1", "Message Data"=w1276) -> (w1279:T4)
            n499 = Enqueue Element(queue=w1281, element=w1279, error in (no error)=w1280) -> (queue out=w1278:refnum<queue>, error out=w1277:errorcluster)  [unwired: 1 in, 1 out]
          }
          frame #2 {
            n500 = for {
              N: 45 -> [w1290]
              i -> [w1289]
              n501 = Subtract(x=w1290, y=w1289) -> (x-y=w1288:i32)
              n502 = Decrement(x=w1288) -> (x-1=→"Target Cal\nFlush Time Remain (sec)":i32)
              n503 = Wait (ms)(milliseconds to wait=u32 1000) -> ()  [unwired: 1 out]
            }
          }
          frame #3 {
            w1294 = TRUE
            n504 = Bundle(cluster=T4 {"Message"="", "Message Data"=variant} ("Message Cluster"), "Message"="V1", "Message Data"=w1294) -> (w1297:T4)
            n505 = local write "V1"(w1294) -> ()
            n506 = Enqueue Element(queue=w1296, element=w1297, error in (no error)=w1295) -> (queue out=w1293:refnum<queue>, error out=w1292:errorcluster)  [unwired: 1 in, 1 out]
          }
          frame #4 {
            n507 = for {
              N: 60 -> [w1306]
              i -> [w1305]
              n508 = Subtract(x=w1306, y=w1305) -> (x-y=w1304:i32)
              n509 = Decrement(x=w1304) -> (x-1=→"Target Cal\nCal Time Remain (sec)":i32)
              n510 = Wait (ms)(milliseconds to wait=u32 1000) -> ()  [unwired: 1 out]
            }
          }
          frame #5 {
            w1314 = FALSE
            n511 = Cluster To Array(cluster=cluster{"Message 3":string, "Message":string} {"Message 3"="V4", "Message"="V1"}) -> (array=w1312:string[])
            n512 = for {
              tunnel: w1312 -> [w1320] mode=indexing
              tunnel: [w1319] -> w1308
              tunnel: [w1318] -> w1309
              tunnel: w1314 -> [w1317]
              tunnel: w1311 -> [w1316]
              tunnel: w1310 -> [w1315]
              n513 = Bundle(cluster=T4 {"Message"="", "Message Data"=variant} ("Message Cluster"), "Message"=w1320, "Message Data"=w1317) -> (w1322:T4)
              n514 = Enqueue Element(queue=w1316, element=w1322, error in (no error)=w1315) -> (queue out=w1319:refnum<queue>, error out=w1318:errorcluster)  [unwired: 1 in, 1 out]
            }
            n515 = local write "V4"(w1314) -> ()
            n516 = local write "V1"(w1314) -> ()
          }
          frame #6 {
            w1324 = 0.0 ("MFC_1\nSLPM Value")
            n517 = local write "MFC_1\nSLPM Value"(w1324) -> ()
            n518 = Bundle(cluster=T4 {"Message"="", "Message Data"=variant} ("Message Cluster"), "Message"="MFC_1", "Message Data"=w1324) -> (w1328:T4)
            n519 = Enqueue Element(queue=w1326, element=w1328, error in (no error)=w1325) -> (error out=w1323:errorcluster)  [unwired: 1 in, 2 out]
          }
          frame #7 {
            n520 = local write "Target Cal"(FALSE ("High Cal")) -> ()
          }
        }
      }
      event "MFC_1\nSLPM Value": Value Change {
        n521 = event-data() -> ()  [unwired: 1 in, 1 out]
        n522 = local read "MFC_1\nSLPM Value"() -> (w1332:dbl)
        n523 = Bundle(cluster=T4 {"Message"="", "Message Data"=variant} ("Message Cluster"), "Message"="MFC_1", "Message Data"=w1332) -> (w1336:T4)
        n524 = Enqueue Element(queue=w1335, element=w1336, error in (no error)=w1334) -> (error out=w1333:errorcluster)  [unwired: 1 in, 2 out]
      }
      event "FGGA UDP Time Offset": Value Change {
        n525 = event-data() -> ("NewVal"=w1339:i32)  [unwired: 1 in, 5 out]
        n526 = Bundle(cluster=T4 {"Message"="", "Message Data"=variant} ("Message Cluster"), "Message"="UDP Time Offset", "Message Data"=w1339) -> (w1343:T4)
        n527 = Enqueue Element(queue=w1342, element=w1343, error in (no error)=w1341) -> (error out=w1340:errorcluster)  [unwired: 1 in, 2 out]
      }
    }
    "FGGA Event Error out" <- w634
  }
  n528 = while {
    shift-right: [w1349] -> _
    shift-left: u8 1 -> [w1350]
    tunnel: w2 -> [w1347]
    tunnel: w1 -> [w1346]
    stop <- FALSE stop-if-true
    # "FGGA pump synchronise to WoW Wait on Wheel Flag"
    n529 = Wait (ms)(milliseconds to wait=u32 1000) -> ()  [unwired: 1 out]
    n530 = case shown="True" "FGGA pump\nsync to WoW" {
      tunnel: [w1353 w1358] -> w1349
      tunnel: w1350 -> [w1353 w1357]
      tunnel: w1347 -> [_ w1356]
      tunnel: w1346 -> [_ w1355]
      frame False {
      }
      frame True {
        n531 = local read "WoW Flag"() -> (w1354:string)
        n532 = Scan Value(string=w1354, format string="%d", default (0 dbl)=u8 0) -> (value=w1358:u8)  [unwired: 1 out]
        n533 = Not Equal?(x=w1358, y=w1357) -> (x != y?=w1361:bool)
        n534 = case shown="True" w1361 {
          tunnel: w1358 -> [_ w1364]
          tunnel: w1356 -> [_ w1363]
          tunnel: w1355 -> [_ w1362]
          frame False {
          }
          frame True {
            n535 = Equal?(x=w1364, y=u8 0) -> (x = y?=w1369:bool)
            n536 = case shown="True" w1369 {
              selector: w1369 -> [w1371 w1372]
              tunnel: [w1371 w1372] -> w1365
              frame False {
              }
              frame True {
              }
            }
            n537 = local write "FGGA Pump"(w1365) -> ()
            n538 = Bundle(cluster=T4 {"Message"="", "Message Data"=variant} ("Message Cluster"), "Message"="FGGA_pump", "Message Data"=w1365) -> (w1366:T4)
            n539 = Enqueue Element(queue=w1363, element=w1366, error in (no error)=w1362) -> ()  [unwired: 1 in, 3 out]
          }
        }
      }
    }
  }
  n540 = Create Network Stream Writer Endpoint(6:w53, 7:10 ("writer buffer size"), 9:w55, 10:"//192.168.101.17/command/reader/FGGA" ("reader url"), 11:"/command/writer/FGGA" ("writer name")) -> (0:w52:errorcluster, 3:w51:refnum<k21>)  [unwired: 2 in]
  n541 = node-c288(w11) -> ()  [unwired: 1 out]
  n542 = while {
    tunnel: w2 -> [w1380]
    shift-right: [w1375] -> _
    shift-left: w51 -> [w1377]
    shift-right: [w1373] -> w48
    shift-left: w52 -> [w1379]
    tunnel: w1 -> [w1374]
    stop <- w1373 stop-if-true
    # "FGGA UI Command Sender"
    n543 = Dequeue Element(queue=w1380, error in (no error)=w1374) -> (element=w1376:T4)  [unwired: 1 in, 3 out]
    n544 = Unbundle By Name(w1376) -> ("Message"=w1378:string)
    n545 = case shown="\"UDP Time Offset\"" w1378 {
      tunnel: w1379 -> [w1381 w1385 w1392 w1399 w1406 w1413 w1420 w1427 w1434 w1441 w1448]
      tunnel: w1377 -> [w1382 w1388 w1395 w1402 w1409 w1416 w1423 w1430 w1437 w1444 w1451]
      tunnel: w1376 -> [_ w1387 w1394 w1401 w1408 w1415 w1422 w1429 w1436 w1443 w1450]
      tunnel: [w1381 w1384 w1391 w1398 w1405 w1412 w1419 w1426 w1433 w1440 w1447] -> w1373
      tunnel: [w1382 w1383 w1390 w1397 w1404 w1411 w1418 w1425 w1432 w1439 w1446] -> w1375
      frame "False", Default {
      }
      frame "V1" {
        n546 = shared-variable-write(w1388, w1385, w1387) -> (w1386:refnum<k21>, w1389:errorcluster)  [unwired: 1 in, 1 out]
        n547 = Flush Stream(8:w1389, 11:w1386) -> (0:w1384:errorcluster, 3:w1383:refnum<k21>)  [unwired: 2 in, 1 out]
      }
      frame "MFC_1" {
        n548 = shared-variable-write(w1395, w1392, w1394) -> (w1393:refnum<k21>, w1396:errorcluster)  [unwired: 1 in, 1 out]
        n549 = Flush Stream(8:w1396, 11:w1393) -> (0:w1391:errorcluster, 3:w1390:refnum<k21>)  [unwired: 2 in, 1 out]
      }
      frame "UDP Time Offset" {
        n550 = shared-variable-write(w1402, w1399, w1401) -> (w1400:refnum<k21>, w1403:errorcluster)  [unwired: 1 in, 1 out]
        n551 = Flush Stream(8:w1403, 11:w1400) -> (0:w1398:errorcluster, 3:w1397:refnum<k21>)  [unwired: 2 in, 1 out]
      }
      frame "V2" {
        n552 = shared-variable-write(w1409, w1406, w1408) -> (w1407:refnum<k21>, w1410:errorcluster)  [unwired: 1 in, 1 out]
        n553 = Flush Stream(8:w1410, 11:w1407) -> (0:w1405:errorcluster, 3:w1404:refnum<k21>)  [unwired: 2 in, 1 out]
      }
      frame "V3" {
        n554 = shared-variable-write(w1416, w1413, w1415) -> (w1414:refnum<k21>, w1417:errorcluster)  [unwired: 1 in, 1 out]
        n555 = Flush Stream(8:w1417, 11:w1414) -> (0:w1412:errorcluster, 3:w1411:refnum<k21>)  [unwired: 2 in, 1 out]
      }
      frame "V4" {
        n556 = shared-variable-write(w1423, w1420, w1422) -> (w1421:refnum<k21>, w1424:errorcluster)  [unwired: 1 in, 1 out]
        n557 = Flush Stream(8:w1424, 11:w1421) -> (0:w1419:errorcluster, 3:w1418:refnum<k21>)  [unwired: 2 in, 1 out]
      }
      frame "FGGA_pump" {
        n558 = shared-variable-write(w1430, w1427, w1429) -> (w1428:refnum<k21>, w1431:errorcluster)  [unwired: 1 in, 1 out]
        n559 = Flush Stream(8:w1431, 11:w1428) -> (0:w1426:errorcluster, 3:w1425:refnum<k21>)  [unwired: 2 in, 1 out]
      }
      frame "Flight Number" {
        n560 = shared-variable-write(w1437, w1434, w1436) -> (w1435:refnum<k21>, w1438:errorcluster)  [unwired: 1 in, 1 out]
        n561 = Flush Stream(8:w1438, 11:w1435) -> (0:w1433:errorcluster, 3:w1432:refnum<k21>)  [unwired: 2 in, 1 out]
      }
      frame "FGGA_restart" {
        n562 = shared-variable-write(w1444, w1441, w1443) -> (w1442:refnum<k21>, w1445:errorcluster)  [unwired: 1 in, 1 out]
        n563 = Flush Stream(8:w1445, 11:w1442) -> (0:w1440:errorcluster, 3:w1439:refnum<k21>)  [unwired: 2 in, 1 out]
      }
      frame "Stop File Write" {
        n564 = shared-variable-write(w1451, w1448, w1450) -> (w1449:refnum<k21>, w1452:errorcluster)  [unwired: 1 in, 1 out]
        n565 = Flush Stream(8:w1452, 11:w1449) -> (0:w1447:errorcluster, 3:w1446:refnum<k21>)  [unwired: 2 in, 1 out]
      }
    }
  }
  "FGGA command sender error out" <- w48
  n566 = Obtain Queue(name (unnamed)="SO2_Command", element data type=w37) -> (queue out=w46:refnum<queue>, error out=w39:errorcluster)  [unwired: 3 in, 1 out]
  n567 = while {
    tunnel: w46 -> [w1456]
    tunnel: w39 -> [w1455]
    tunnel: [w1453] -> _
    stop <- FALSE stop-if-true
    # "SO2 UI Event Handler Loop"
    n568 = event shown="[2] \"SO2 Zeroing\": Value Change" {
      selector: _ -> [_ _ _ _ _ _ _ _ _ _ _ _ _ _ _ _ _ _]
      dyn-events: _ -> [_ _ _ _ _ _ _ _ _ _ _ _ _ _ _ _ _ _]
      timeout: _ -> [_ _ _ _ _ _ _ _ _ _ _ _ _ _ _ _ _ _]
      tunnel: w1456 -> [w1463 w1471 w1504 w1543 w1612 w1619 w1623 w1630 w1637 w1644 w1651 w1658 w1665 w1672 w1679 w1686 w1693 w1700]
      tunnel: w1455 -> [w1462 w1470 w1503 w1542 w1611 w1618 w1622 w1629 w1636 w1643 w1650 w1657 w1664 w1671 w1678 w1685 w1692 w1699]
      tunnel: [w1457 w1469 w1502 _ w1606 w1613 w1621 w1628 w1635 w1642 w1649 w1656 w1663 w1670 w1677 w1684 w1691 w1698] -> w1453
      event "V9": Value Change {
        n569 = event-data() -> ("NewVal"=w1460:bool)  [unwired: 1 in]
        n570 = Bundle(cluster=T4 {"Message"="", "Message Data"=variant} ("Message Cluster"), "Message"="V9", "Message Data"=w1460) -> (w1458:T4)
        n571 = Enqueue Element(queue=w1463, element=w1458, error in (no error)=w1462) -> (error out=w1457:errorcluster)  [unwired: 1 in, 2 out]
      }
      event "SO2 Flush": Value Change {
        n572 = event-data() -> ()  [unwired: 1 in, 1 out]
        n573 = flat-sequence {
          tunnel: w1471 -> [w1479]
          tunnel: w1470 -> [w1478]
          tunnel: [w1474] -> w1468
          tunnel: [w1472] -> w1464
          tunnel: w1468 -> [w1482]
          tunnel: [w1482] -> w1467
          tunnel: [w1480] -> w1465
          tunnel: w1464 -> [w1480]
          tunnel: w1467 -> [w1490]
          tunnel: [w1489] -> w1466
          tunnel: w1465 -> [w1491]
          tunnel: [w1496] -> w1469
          tunnel: w1466 -> [w1496]
          frame #0 {
            w1473 = TRUE ("SO2 Flush")
            n574 = Bundle(cluster=T4 {"Message"="", "Message Data"=variant} ("Message Cluster"), "Message"="V9", "Message Data"=w1473) -> (w1475:T4)
            n575 = local write "V9"(w1473) -> ()
            n576 = Enqueue Element(queue=w1479, element=w1475, error in (no error)=w1478) -> (queue out=w1472:refnum<queue>, error out=w1474:errorcluster)  [unwired: 1 in, 1 out]
          }
          frame #1 {
            n577 = for {
              N: 15 -> [w1486]
              i -> [w1485]
              n578 = Subtract(x=w1486, y=w1485) -> (x-y=w1484:i32)
              n579 = Decrement(x=w1484) -> (x-1=w1483:i32)
              n580 = local write "SO2 Flush\nTime Remain (sec)"(w1483) -> ()
              n581 = Wait (ms)(milliseconds to wait=u32 1000) -> ()  [unwired: 1 out]
            }
          }
          frame #2 {
            w1488 = FALSE
            n582 = Bundle(cluster=T4 {"Message"="", "Message Data"=variant} ("Message Cluster"), "Message"="V9", "Message Data"=w1488) -> (w1492:T4)
            n583 = local write "V9"(w1488) -> ()
            n584 = Enqueue Element(queue=w1491, element=w1492, error in (no error)=w1490) -> (error out=w1489:errorcluster)  [unwired: 1 in, 2 out]
          }
          frame #3 {
            n585 = local write "SO2 Flush"(FALSE ("SO2 Flush")) -> ()
          }
        }
      }
      event "SO2 Zeroing": Value Change {
        n586 = event-data() -> ()  [unwired: 1 in, 1 out]
        n587 = flat-sequence {
          tunnel: w1504 -> [w1512]
          tunnel: w1503 -> [w1511]
          tunnel: [w1507] -> w1501
          tunnel: [w1505] -> w1497
          tunnel: w1501 -> [w1515]
          tunnel: [w1515] -> w1500
          tunnel: [w1513] -> w1498
          tunnel: w1497 -> [w1513]
          tunnel: w1500 -> [w1523]
          tunnel: [w1522] -> w1499
          tunnel: w1498 -> [w1524]
          tunnel: [w1529] -> w1502
          tunnel: w1499 -> [w1529]
          frame #0 {
            w1506 = TRUE ("SO2 Flush")
            n588 = local write "SO2 V6"(w1506) -> ()
            n589 = Bundle(cluster=T4 {"Message"="", "Message Data"=variant} ("Message Cluster"), "Message"="V6", "Message Data"=w1506) -> (w1508:T4)
            n590 = Enqueue Element(queue=w1512, element=w1508, error in (no error)=w1511) -> (queue out=w1505:refnum<queue>, error out=w1507:errorcluster)  [unwired: 1 in, 1 out]
          }
          frame #1 {
            # "10 Mins Count down"
            n591 = for {
              N: 600 -> [w1519]
              i -> [w1518]
              n592 = Subtract(x=w1519, y=w1518) -> (x-y=w1517:i32)
              n593 = Decrement(x=w1517) -> (x-1=w1516:i32)
              n594 = local write "SO2 Zeroing\nTime Remain (sec)"(w1516) -> ()
              n595 = Wait (ms)(milliseconds to wait=u32 1000) -> ()  [unwired: 1 out]
            }
          }
          frame #2 {
            w1521 = FALSE
            n596 = Bundle(cluster=T4 {"Message"="", "Message Data"=variant} ("Message Cluster"), "Message"="V6", "Message Data"=w1521) -> (w1525:T4)
            n597 = local write "SO2 V6"(w1521) -> ()
            n598 = Enqueue Element(queue=w1524, element=w1525, error in (no error)=w1523) -> (error out=w1522:errorcluster)  [unwired: 1 in, 2 out]
          }
          frame #3 {
            n599 = local write "SO2 Zeroing"(FALSE ("SO2 Flush")) -> ()
          }
        }
      }
      event "SO2 CAL": Value Change {
        n600 = event-data() -> ()  [unwired: 1 in, 1 out]
        n601 = flat-sequence {
          tunnel: w1543 -> [w1551]
          tunnel: w1542 -> [w1550]
          tunnel: [w1546] -> w1541
          tunnel: [w1545] -> w1539
          tunnel: w1541 -> [w1555]
          tunnel: [w1554] -> w1540
          tunnel: w1539 -> [w1556]
          tunnel: [w1552] -> w1537
          tunnel: w1540 -> [w1562]
          tunnel: [w1562] -> w1538
          tunnel: w1537 -> [w1560]
          tunnel: [w1560] -> w1536
          tunnel: w1538 -> [w1571]
          tunnel: w1536 -> [w1572]
          tunnel: [w1569] -> w1534
          tunnel: [w1568] -> w1532
          tunnel: [w1577] -> w1535
          tunnel: w1534 -> [w1577]
          tunnel: [w1576] -> w1533
          tunnel: w1532 -> [w1576]
          tunnel: w1535 -> [w1587]
          tunnel: w1533 -> [w1586]
          tunnel: [w1585] -> w1531
          tunnel: [w1584] -> w1530
          tunnel: w1531 -> [w1601]
          tunnel: w1530 -> [w1600]
          frame #0 {
            w1544 = TRUE ("SO2 Flush")
            n602 = Bundle(cluster=T4 {"Message"="", "Message Data"=variant} ("Message Cluster"), "Message"="V9", "Message Data"=w1544) -> (w1547:T4)
            n603 = local write "V9"(w1544) -> ()
            n604 = Enqueue Element(queue=w1551, element=w1547, error in (no error)=w1550) -> (queue out=w1545:refnum<queue>, error out=w1546:errorcluster)  [unwired: 1 in, 1 out]
          }
          frame #1 {
            n605 = local read "MFC_2 User Set Value"() -> (w1553:dbl)
            n606 = local write "MFC_2\nSLPM Value"(w1553) -> ()
            n607 = Bundle(cluster=T4 {"Message"="", "Message Data"=variant} ("Message Cluster"), "Message"="MFC_2", "Message Data"=w1553) -> (w1557:T4)
            n608 = Enqueue Element(queue=w1556, element=w1557, error in (no error)=w1555) -> (queue out=w1552:refnum<queue>, error out=w1554:errorcluster)  [unwired: 1 in, 1 out]
          }
          frame #2 {
            n609 = for {
              N: 45 -> [w1566]
              i -> [w1565]
              n610 = Subtract(x=w1566, y=w1565) -> (x-y=w1564:i32)
              n611 = Decrement(x=w1564) -> (x-1=w1563:i32)
              n612 = local write "SO2 Flush\nTime Remain (sec)"(w1563) -> ()
              n613 = Wait (ms)(milliseconds to wait=u32 1000) -> ()  [unwired: 1 out]
            }
          }
          frame #3 {
            w1570 = TRUE ("SO2 Flush")
            n614 = Bundle(cluster=T4 {"Message"="", "Message Data"=variant} ("Message Cluster"), "Message"="V8", "Message Data"=w1570) -> (w1573:T4)
            n615 = local write "V8"(w1570) -> ()
            n616 = Enqueue Element(queue=w1572, element=w1573, error in (no error)=w1571) -> (queue out=w1569:refnum<queue>, error out=w1568:errorcluster)  [unwired: 1 in, 1 out]
          }
          frame #4 {
            n617 = for {
              N: 60 -> [w1582]
              i -> [w1581]
              n618 = Subtract(x=w1582, y=w1581) -> (x-y=w1580:i32)
              n619 = Decrement(x=w1580) -> (x-1=w1579:i32)
              n620 = local write "SO2 CAL\nTime Remain (sec)"(w1579) -> ()
              n621 = Wait (ms)(milliseconds to wait=u32 1000) -> ()  [unwired: 1 out]
            }
          }
          frame #5 {
            n622 = Cluster To Array(cluster=cluster{"Message":string, "Message 2":string} {"Message"="V8", "Message 2"="V9"}) -> (array=w1589:string[])
            n623 = for {
              tunnel: w1589 -> [w1596] mode=indexing
              tunnel: FALSE ("SO2 Flush") -> [w1595]
              tunnel: w1587 -> [w1594]
              tunnel: w1586 -> [w1593]
              tunnel: [w1592] -> w1585
              tunnel: [w1591] -> w1584
              n624 = Bundle(cluster=T4 {"Message"="", "Message Data"=variant} ("Message Cluster"), "Message"=w1596, "Message Data"=w1595) -> (w1597:T4)
              n625 = Enqueue Element(queue=w1594, element=w1597, error in (no error)=w1593) -> (queue out=w1592:refnum<queue>, error out=w1591:errorcluster)  [unwired: 1 in, 1 out]
            }
          }
          frame #6 {
            w1599 = 0.0 ("MFC_2\nSLPM Value")
            n626 = local write "MFC_2\nSLPM Value"(w1599) -> ()
            n627 = Bundle(cluster=T4 {"Message"="", "Message Data"=variant} ("Message Cluster"), "Message"="MFC_2", "Message Data"=w1599) -> (w1602:T4)
            n628 = Enqueue Element(queue=w1601, element=w1602, error in (no error)=w1600) -> ()  [unwired: 1 in, 3 out]
          }
          frame #7 {
            w1605 = FALSE ("SO2 Flush")
            n629 = local write "SO2 CAL"(w1605) -> ()
            n630 = local write "V9"(w1605) -> ()
            n631 = local write "V8"(w1605) -> ()
          }
        }
      }
      event "MFC_2\nSLPM Value": Value Change {
        n632 = event-data() -> ("NewVal"=w1609:dbl)  [unwired: 1 in]
        n633 = Bundle(cluster=T4 {"Message"="", "Message Data"=variant} ("Message Cluster"), "Message"="MFC_2", "Message Data"=w1609) -> (w1607:T4)
        n634 = Enqueue Element(queue=w1612, element=w1607, error in (no error)=w1611) -> (error out=w1606:errorcluster)  [unwired: 1 in, 2 out]
      }
      event "MFC_3\nSLPM Value": Value Change {
        n635 = event-data() -> ("NewVal"=w1616:dbl)  [unwired: 1 in]
        n636 = Bundle(cluster=T4 {"Message"="", "Message Data"=variant} ("Message Cluster"), "Message"="MFC_3", "Message Data"=w1616) -> (w1614:T4)
        n637 = Enqueue Element(queue=w1619, element=w1614, error in (no error)=w1618) -> (error out=w1613:errorcluster)  [unwired: 1 in, 2 out]
      }
      event "V8": Value Change {
        n638 = event-data() -> ("NewVal"=w1620:bool)  [unwired: 1 in]
        n639 = Bundle(cluster=T4 {"Message"="", "Message Data"=variant} ("Message Cluster"), "Message"="V8", "Message Data"=w1620) -> (w1624:T4)
        n640 = Enqueue Element(queue=w1623, element=w1624, error in (no error)=w1622) -> (error out=w1621:errorcluster)  [unwired: 1 in, 2 out]
      }
      event "SO2 V6": Value Change {
        n641 = event-data() -> ("NewVal"=w1627:bool)  [unwired: 1 in]
        n642 = Bundle(cluster=T4 {"Message"="", "Message Data"=variant} ("Message Cluster"), "Message"="V6", "Message Data"=w1627) -> (w1631:T4)
        n643 = Enqueue Element(queue=w1630, element=w1631, error in (no error)=w1629) -> (error out=w1628:errorcluster)  [unwired: 1 in, 2 out]
      }
      event "Simulate Conc": Value Change {
        n644 = event-data() -> ("NewVal"=w1634:bool)  [unwired: 1 in]
        n645 = Bundle(cluster=T4 {"Message"="", "Message Data"=variant} ("Message Cluster"), "Message"="Simulate Conc", "Message Data"=w1634) -> (w1638:T4)
        n646 = Enqueue Element(queue=w1637, element=w1638, error in (no error)=w1636) -> (error out=w1635:errorcluster)  [unwired: 1 in, 2 out]
      }
      event "SO2 UDP Time Offset": Value Change {
        n647 = event-data() -> ("NewVal"=w1641:i32)  [unwired: 1 in]
        n648 = Bundle(cluster=T4 {"Message"="", "Message Data"=variant} ("Message Cluster"), "Message"="UDP Time Offset", "Message Data"=w1641) -> (w1645:T4)
        n649 = Enqueue Element(queue=w1644, element=w1645, error in (no error)=w1643) -> (error out=w1642:errorcluster)  [unwired: 1 in, 2 out]
      }
      event "Simulate STEL Conc": Value Change {
        n650 = event-data() -> ("NewVal"=w1648:dbl)  [unwired: 1 in]
        n651 = Bundle(cluster=T4 {"Message"="", "Message Data"=variant} ("Message Cluster"), "Message"="Simulate STEL Conc", "Message Data"=w1648) -> (w1652:T4)
        n652 = Enqueue Element(queue=w1651, element=w1652, error in (no error)=w1650) -> (error out=w1649:errorcluster)  [unwired: 1 in, 2 out]
      }
      event "Simulate TWA Conc": Value Change {
        n653 = event-data() -> ("NewVal"=w1655:dbl)  [unwired: 1 in]
        n654 = Bundle(cluster=T4 {"Message"="", "Message Data"=variant} ("Message Cluster"), "Message"="Simulate TWA Conc", "Message Data"=w1655) -> (w1659:T4)
        n655 = Enqueue Element(queue=w1658, element=w1659, error in (no error)=w1657) -> (error out=w1656:errorcluster)  [unwired: 1 in, 2 out]
      }
      event "10mins STEL Limit": Value Change {
        n656 = event-data() -> ("NewVal"=w1662:i32)  [unwired: 1 in]
        n657 = Bundle(cluster=T4 {"Message"="", "Message Data"=variant} ("Message Cluster"), "Message"="10mins STEL Limit", "Message Data"=w1662) -> (w1666:T4)
        n658 = Enqueue Element(queue=w1665, element=w1666, error in (no error)=w1664) -> (error out=w1663:errorcluster)  [unwired: 1 in, 2 out]
      }
      event "8hr TWA Limit": Value Change {
        n659 = event-data() -> ("NewVal"=w1669:i32)  [unwired: 1 in]
        n660 = Bundle(cluster=T4 {"Message"="", "Message Data"=variant} ("Message Cluster"), "Message"="8hr TWA Limit", "Message Data"=w1669) -> (w1673:T4)
        n661 = Enqueue Element(queue=w1672, element=w1673, error in (no error)=w1671) -> (error out=w1670:errorcluster)  [unwired: 1 in, 2 out]
      }
      event "SO2 Offset": Value Change {
        n662 = event-data() -> ("NewVal"=w1676:dbl)  [unwired: 1 in]
        n663 = Bundle(cluster=T4 {"Message"="", "Message Data"=variant} ("Message Cluster"), "Message"="Offset", "Message Data"=w1676) -> (w1680:T4)
        n664 = Enqueue Element(queue=w1679, element=w1680, error in (no error)=w1678) -> (error out=w1677:errorcluster)  [unwired: 1 in, 2 out]
      }
      event "SO2 Slope": Value Change {
        n665 = event-data() -> ("NewVal"=w1683:dbl)  [unwired: 1 in]
        n666 = Bundle(cluster=T4 {"Message"="", "Message Data"=variant} ("Message Cluster"), "Message"="Slope", "Message Data"=w1683) -> (w1687:T4)
        n667 = Enqueue Element(queue=w1686, element=w1687, error in (no error)=w1685) -> (error out=w1684:errorcluster)  [unwired: 1 in, 2 out]
      }
      event "Confirm Flight Number": Value Change {
        n668 = event-data() -> ()  [unwired: 1 in, 6 out]
        n669 = local read "Flight Number"() -> (w1690:string)
        n670 = Bundle(cluster=T4 {"Message"="", "Message Data"=variant} ("Message Cluster"), "Message"="Flight Number", "Message Data"=w1690) -> (w1694:T4)
        n671 = Enqueue Element(queue=w1693, element=w1694, error in (no error)=w1692) -> (error out=w1691:errorcluster)  [unwired: 1 in, 2 out]
      }
      event "cRIO File IO Stop\n(USB Flash Drive Unmount)": Value Change {
        n672 = event-data() -> ("NewVal"=w1697:bool)  [unwired: 1 in]
        n673 = Bundle(cluster=T4 {"Message"="", "Message Data"=variant} ("Message Cluster"), "Message"="Stop File Write", "Message Data"=w1697) -> (w1701:T4)
        n674 = Enqueue Element(queue=w1700, element=w1701, error in (no error)=w1699) -> (error out=w1698:errorcluster)  [unwired: 1 in, 2 out]
      }
    }
    "SO2 Event error out" <- w1453
  }
  n675 = Create Network Stream Writer Endpoint(6:w43, 7:10 ("writer buffer size"), 9:w37, 10:"//192.168.101.17/command/reader/SO2" ("reader url"), 11:"/command/writer/SO2" ("writer name")) -> (0:w42:errorcluster, 3:w41:refnum<k21>)  [unwired: 2 in]
  n676 = while {
    tunnel: w46 -> [w1711]
    shift-right: [w1706] -> _
    shift-left: w41 -> [w1708]
    shift-right: [w1704] -> w38
    shift-left: w42 -> [w1710]
    tunnel: w39 -> [w1705]
    stop <- w1704 stop-if-true
    # "SO2 UI Command Sender"
    n677 = Dequeue Element(queue=w1711, error in (no error)=w1705) -> (element=w1707:T4)  [unwired: 1 in, 3 out]
    n678 = Unbundle By Name(w1707) -> ("Message"=w1709:string)
    n679 = case shown="\"UDP Time Offset\"" w1709 {
      tunnel: w1710 -> [w1712 w1716 w1723 w1730 w1737 w1744 w1751 w1758 w1765 w1772 w1779 w1786 w1793 w1800 w1807 w1814]
      tunnel: w1708 -> [w1713 w1719 w1726 w1733 w1740 w1747 w1754 w1761 w1768 w1775 w1782 w1789 w1796 w1803 w1810 w1817]
      tunnel: w1707 -> [_ w1718 w1725 w1732 w1739 w1746 w1753 w1760 w1767 w1774 w1781 w1788 w1795 w1802 w1809 w1816]
      tunnel: [w1712 w1715 w1722 w1729 w1736 w1743 w1750 w1757 w1764 w1771 w1778 w1785 w1792 w1799 w1806 w1813] -> w1704
      tunnel: [w1713 w1714 w1721 w1728 w1735 w1742 w1749 w1756 w1763 w1770 w1777 w1784 w1791 w1798 w1805 w1812] -> w1706
      frame "False", Default {
      }
      frame "V9" {
        n680 = shared-variable-write(w1719, w1716, w1718) -> (w1717:refnum<k21>, w1720:errorcluster)  [unwired: 1 in, 1 out]
        n681 = Flush Stream(8:w1720, 11:w1717) -> (0:w1715:errorcluster, 3:w1714:refnum<k21>)  [unwired: 2 in, 1 out]
      }
      frame "MFC_2" {
        n682 = shared-variable-write(w1726, w1723, w1725) -> (w1724:refnum<k21>, w1727:errorcluster)  [unwired: 1 in, 1 out]
        n683 = Flush Stream(8:w1727, 11:w1724) -> (0:w1722:errorcluster, 3:w1721:refnum<k21>)  [unwired: 2 in, 1 out]
      }
      frame "MFC_3" {
        n684 = shared-variable-write(w1733, w1730, w1732) -> (w1731:refnum<k21>, w1734:errorcluster)  [unwired: 1 in, 1 out]
        n685 = Flush Stream(8:w1734, 11:w1731) -> (0:w1729:errorcluster, 3:w1728:refnum<k21>)  [unwired: 2 in, 1 out]
      }
      frame "V6" {
        n686 = shared-variable-write(w1740, w1737, w1739) -> (w1738:refnum<k21>, w1741:errorcluster)  [unwired: 1 in, 1 out]
        n687 = Flush Stream(8:w1741, 11:w1738) -> (0:w1736:errorcluster, 3:w1735:refnum<k21>)  [unwired: 2 in, 1 out]
      }
      frame "Simulate Conc" {
        n688 = shared-variable-write(w1747, w1744, w1746) -> (w1745:refnum<k21>, w1748:errorcluster)  [unwired: 1 in, 1 out]
        n689 = Flush Stream(8:w1748, 11:w1745) -> (0:w1743:errorcluster, 3:w1742:refnum<k21>)  [unwired: 2 in, 1 out]
      }
      frame "Simulate STEL Conc" {
        n690 = shared-variable-write(w1754, w1751, w1753) -> (w1752:refnum<k21>, w1755:errorcluster)  [unwired: 1 in, 1 out]
        n691 = Flush Stream(8:w1755, 11:w1752) -> (0:w1750:errorcluster, 3:w1749:refnum<k21>)  [unwired: 2 in, 1 out]
      }
      frame "Simulate TWA Conc" {
        n692 = shared-variable-write(w1761, w1758, w1760) -> (w1759:refnum<k21>, w1762:errorcluster)  [unwired: 1 in, 1 out]
        n693 = Flush Stream(8:w1762, 11:w1759) -> (0:w1757:errorcluster, 3:w1756:refnum<k21>)  [unwired: 2 in, 1 out]
      }
      frame "10mins STEL Limit" {
        n694 = shared-variable-write(w1768, w1765, w1767) -> (w1766:refnum<k21>, w1769:errorcluster)  [unwired: 1 in, 1 out]
        n695 = Flush Stream(8:w1769, 11:w1766) -> (0:w1764:errorcluster, 3:w1763:refnum<k21>)  [unwired: 2 in, 1 out]
      }
      frame "8hr TWA Limit" {
        n696 = shared-variable-write(w1775, w1772, w1774) -> (w1773:refnum<k21>, w1776:errorcluster)  [unwired: 1 in, 1 out]
        n697 = Flush Stream(8:w1776, 11:w1773) -> (0:w1771:errorcluster, 3:w1770:refnum<k21>)  [unwired: 2 in, 1 out]
      }
      frame "Offset" {
        n698 = shared-variable-write(w1782, w1779, w1781) -> (w1780:refnum<k21>, w1783:errorcluster)  [unwired: 1 in, 1 out]
        n699 = Flush Stream(8:w1783, 11:w1780) -> (0:w1778:errorcluster, 3:w1777:refnum<k21>)  [unwired: 2 in, 1 out]
      }
      frame "Slope" {
        n700 = shared-variable-write(w1789, w1786, w1788) -> (w1787:refnum<k21>, w1790:errorcluster)  [unwired: 1 in, 1 out]
        n701 = Flush Stream(8:w1790, 11:w1787) -> (0:w1785:errorcluster, 3:w1784:refnum<k21>)  [unwired: 2 in, 1 out]
      }
      frame "Flight Number" {
        n702 = shared-variable-write(w1796, w1793, w1795) -> (w1794:refnum<k21>, w1797:errorcluster)  [unwired: 1 in, 1 out]
        n703 = Flush Stream(8:w1797, 11:w1794) -> (0:w1792:errorcluster, 3:w1791:refnum<k21>)  [unwired: 2 in, 1 out]
      }
      frame "Stop File Write" {
        n704 = shared-variable-write(w1803, w1800, w1802) -> (w1801:refnum<k21>, w1804:errorcluster)  [unwired: 1 in, 1 out]
        n705 = Flush Stream(8:w1804, 11:w1801) -> (0:w1799:errorcluster, 3:w1798:refnum<k21>)  [unwired: 2 in, 1 out]
      }
      frame "UDP Time Offset" {
        n706 = shared-variable-write(w1810, w1807, w1809) -> (w1808:refnum<k21>, w1811:errorcluster)  [unwired: 1 in, 1 out]
        n707 = Flush Stream(8:w1811, 11:w1808) -> (0:w1806:errorcluster, 3:w1805:refnum<k21>)  [unwired: 2 in, 1 out]
      }
      frame "V8" {
        n708 = shared-variable-write(w1817, w1814, w1816) -> (w1815:refnum<k21>, w1818:errorcluster)  [unwired: 1 in, 1 out]
        n709 = Flush Stream(8:w1818, 11:w1815) -> (0:w1813:errorcluster, 3:w1812:refnum<k21>)  [unwired: 2 in, 1 out]
      }
    }
  }
  "SO2 command sender error out" <- w38
  n710 = Obtain Queue(name (unnamed)="TEi43c_Command", element data type=w26) -> (queue out=w35:refnum<queue>, error out=w28:errorcluster)  [unwired: 3 in, 1 out]
  n711 = Create Network Stream Writer Endpoint(6:w32, 7:10 ("writer buffer size"), 9:w26, 10:"//192.168.101.17/command/reader/TEi43c" ("reader url"), 11:"/command/writer/TEi43c" ("writer name")) -> (0:w31:errorcluster, 3:w30:refnum<k21>)  [unwired: 2 in]
  n712 = while {
    tunnel: w35 -> [w1822]
    tunnel: w28 -> [w1821]
    tunnel: [w1819] -> _
    stop <- FALSE stop-if-true
    # "TEi43c Ozone UI Event Handler Loop"
    n713 = event shown="[0] \"Ozone Zeroing\": Value Change" {
      selector: _ -> [_ _ _ _ _]
      dyn-events: _ -> [_ _ _ _ _]
      timeout: _ -> [_ _ _ _ _]
      tunnel: w1822 -> [w1830 w1858 w1866 w1873 w1880]
      tunnel: w1821 -> [w1829 w1857 w1865 w1872 w1879]
      tunnel: [w1828 w1856 w1864 w1871 w1878] -> w1819
      event "Ozone Zeroing": Value Change {
        n714 = event-data() -> ()  [unwired: 1 in, 6 out]
        n715 = flat-sequence {
          tunnel: w1830 -> [w1835]
          tunnel: w1829 -> [w1834]
          tunnel: [w1833] -> w1827
          tunnel: [w1831] -> w1823
          tunnel: w1827 -> [w1841]
          tunnel: [w1841] -> w1826
          tunnel: [w1839] -> w1824
          tunnel: w1823 -> [w1839]
          tunnel: w1826 -> [w1849]
          tunnel: [w1848] -> w1825
          tunnel: w1824 -> [w1850]
          tunnel: [w1855] -> w1828
          tunnel: w1825 -> [w1855]
          frame #0 {
            w1832 = TRUE
            n716 = local write "Ozone V6"(w1832) -> ()
            n717 = Bundle(cluster=T4 {"Message"="", "Message Data"=variant} ("Message Cluster"), "Message"="V6", "Message Data"=w1832) -> (w1836:T4)
            n718 = Enqueue Element(queue=w1835, element=w1836, error in (no error)=w1834) -> (queue out=w1831:refnum<queue>, error out=w1833:errorcluster)  [unwired: 1 in, 1 out]
          }
          frame #1 {
            # "10 Mins Count down"
            n719 = for {
              N: 600 -> [w1845]
              i -> [w1844]
              n720 = Subtract(x=w1845, y=w1844) -> (x-y=w1843:i32)
              n721 = Decrement(x=w1843) -> (x-1=→"Ozone Zeroing\nTime Remain (sec)":i32)
              n722 = Wait (ms)(milliseconds to wait=u32 1000) -> ()  [unwired: 1 out]
            }
          }
          frame #2 {
            w1847 = FALSE
            n723 = local write "Ozone V6"(w1847) -> ()
            n724 = Bundle(cluster=T4 {"Message"="", "Message Data"=variant} ("Message Cluster"), "Message"="V6", "Message Data"=w1847) -> (w1851:T4)
            n725 = Enqueue Element(queue=w1850, element=w1851, error in (no error)=w1849) -> (error out=w1848:errorcluster)  [unwired: 1 in, 2 out]
          }
          frame #3 {
            n726 = local write "Ozone Zeroing"(FALSE ("Ozone Zeroing")) -> ()
          }
        }
      }
      event "Ozone V6": Value Change {
        n727 = event-data() -> ("NewVal"=w1859:bool)  [unwired: 1 in]
        n728 = Bundle(cluster=T4 {"Message"="", "Message Data"=variant} ("Message Cluster"), "Message"="V6", "Message Data"=w1859) -> (w1860:T4)
        n729 = Enqueue Element(queue=w1858, element=w1860, error in (no error)=w1857) -> (error out=w1856:errorcluster)  [unwired: 1 in, 2 out]
      }
      event "cRIO File IO Stop\n(USB Flash Drive Unmount)": Value Change {
        n730 = event-data() -> ("NewVal"=w1863:bool)  [unwired: 1 in]
        n731 = Bundle(cluster=T4 {"Message"="", "Message Data"=variant} ("Message Cluster"), "Message"="Stop File Write", "Message Data"=w1863) -> (w1867:T4)
        n732 = Enqueue Element(queue=w1866, element=w1867, error in (no error)=w1865) -> (error out=w1864:errorcluster)  [unwired: 1 in, 2 out]
      }
      event "Ozone UDP Time Offset": Value Change {
        n733 = event-data() -> ("NewVal"=w1870:i32)  [unwired: 1 in]
        n734 = Bundle(cluster=T4 {"Message"="", "Message Data"=variant} ("Message Cluster"), "Message"="UDP Time Offset", "Message Data"=w1870) -> (w1874:T4)
        n735 = Enqueue Element(queue=w1873, element=w1874, error in (no error)=w1872) -> (error out=w1871:errorcluster)  [unwired: 1 in, 2 out]
      }
      event "Confirm Flight Number": Value Change {
        n736 = event-data() -> ()  [unwired: 1 in, 5 out]
        n737 = local read "Flight Number"() -> (w1877:string)
        n738 = Bundle(cluster=T4 {"Message"="", "Message Data"=variant} ("Message Cluster"), "Message"="Flight Number", "Message Data"=w1877) -> (w1881:T4)
        n739 = Enqueue Element(queue=w1880, element=w1881, error in (no error)=w1879) -> (error out=w1878:errorcluster)  [unwired: 1 in, 2 out]
      }
    }
    "Ozone Event error out" <- w1819
  }
  n740 = while {
    tunnel: w35 -> [w1891]
    shift-right: [w1886] -> _
    shift-left: w30 -> [w1888]
    shift-right: [w1884] -> w27
    shift-left: w31 -> [w1890]
    tunnel: w28 -> [w1885]
    stop <- w1884 stop-if-true
    # "TEi43c Ozone UI Command Sender"
    n741 = Dequeue Element(queue=w1891, error in (no error)=w1885) -> (element=w1887:T4)  [unwired: 1 in, 3 out]
    n742 = Unbundle By Name(w1887) -> ("Message"=w1889:string)
    n743 = case shown="\"UDP Time Offset\"" w1889 {
      tunnel: w1890 -> [w1892 w1896 w1903 w1910 w1917]
      tunnel: w1888 -> [w1893 w1899 w1906 w1913 w1920]
      tunnel: w1887 -> [_ w1898 w1905 w1912 w1919]
      tunnel: [w1892 w1895 w1902 w1909 w1916] -> w1884
      tunnel: [w1893 w1894 w1901 w1908 w1915] -> w1886
      frame "False", Default {
      }
      frame "V6" {
        n744 = shared-variable-write(w1899, w1896, w1898) -> (w1897:refnum<k21>, w1900:errorcluster)  [unwired: 1 in, 1 out]
        n745 = Flush Stream(8:w1900, 11:w1897) -> (0:w1895:errorcluster, 3:w1894:refnum<k21>)  [unwired: 2 in, 1 out]
      }
      frame "Stop File Write" {
        n746 = shared-variable-write(w1906, w1903, w1905) -> (w1904:refnum<k21>, w1907:errorcluster)  [unwired: 1 in, 1 out]
        n747 = Flush Stream(8:w1907, 11:w1904) -> (0:w1902:errorcluster, 3:w1901:refnum<k21>)  [unwired: 2 in, 1 out]
      }
      frame "Flight Number" {
        n748 = shared-variable-write(w1913, w1910, w1912) -> (w1911:refnum<k21>, w1914:errorcluster)  [unwired: 1 in, 1 out]
        n749 = Flush Stream(8:w1914, 11:w1911) -> (0:w1909:errorcluster, 3:w1908:refnum<k21>)  [unwired: 2 in, 1 out]
      }
      frame "UDP Time Offset" {
        n750 = shared-variable-write(w1920, w1917, w1919) -> (w1918:refnum<k21>, w1921:errorcluster)  [unwired: 1 in, 1 out]
        n751 = Flush Stream(8:w1921, 11:w1918) -> (0:w1916:errorcluster, 3:w1915:refnum<k21>)  [unwired: 2 in, 1 out]
      }
    }
  }
  "Ozone command sender error out" <- w27
  n752 = Obtain Queue(name (unnamed)="2BOzone_Command", element data type=w14) -> (queue out=w23:refnum<queue>, error out=w16:errorcluster)  [unwired: 3 in, 1 out]
  n753 = Create Network Stream Writer Endpoint(6:w20, 7:10 ("writer buffer size"), 9:w14, 10:"//192.168.101.17/command/reader/2BOzone" ("reader url"), 11:"/command/writer/2BOzone" ("writer name")) -> (0:w19:errorcluster, 3:w18:refnum<k21>)  [unwired: 2 in]
  n754 = while {
    tunnel: w23 -> [w1925]
    tunnel: w16 -> [w1924]
    tunnel: [w1922] -> _
    stop <- FALSE stop-if-true
    # "2BOzone UI Event Handler Loop"
    n755 = event shown="[7] \"Confirm Flight Number\": Value Change" {
      selector: _ -> [_ _ _ _ _ _ _ _]
      dyn-events: _ -> [_ _ _ _ _ _ _ _]
      timeout: _ -> [_ _ _ _ _ _ _ _]
      tunnel: w1925 -> [w1929 w1936 w1943 w1950 w1957 w1964 w1971 w1978]
      tunnel: w1924 -> [w1928 w1935 w1942 w1949 w1956 w1963 w1970 w1977]
      tunnel: [w1927 w1934 w1941 w1948 w1955 w1962 w1969 w1976] -> w1922
      event "Ambient = OFF\nCabin = ON": Value Change {
        n756 = event-data() -> ("NewVal"=w1926:bool)  [unwired: 1 in]
        n757 = Bundle(cluster=T4 {"Message"="", "Message Data"=variant} ("Message Cluster"), "Message"="Ambient/Cabin", "Message Data"=w1926) -> (w1930:T4)
        n758 = Enqueue Element(queue=w1929, element=w1930, error in (no error)=w1928) -> (error out=w1927:errorcluster)  [unwired: 1 in, 2 out]
      }
      event "Simulate 2B Conc": Value Change {
        n759 = event-data() -> ("NewVal"=w1933:bool)  [unwired: 1 in]
        n760 = Bundle(cluster=T4 {"Message"="", "Message Data"=variant} ("Message Cluster"), "Message"="Simulate_conc", "Message Data"=w1933) -> (w1937:T4)
        n761 = Enqueue Element(queue=w1936, element=w1937, error in (no error)=w1935) -> (error out=w1934:errorcluster)  [unwired: 1 in, 2 out]
      }
      event "Simulate Inst Conc": Value Change {
        n762 = event-data() -> ("NewVal"=w1940:i32)  [unwired: 1 in]
        n763 = Bundle(cluster=T4 {"Message"="", "Message Data"=variant} ("Message Cluster"), "Message"="Simulate_inst_conc", "Message Data"=w1940) -> (w1944:T4)
        n764 = Enqueue Element(queue=w1943, element=w1944, error in (no error)=w1942) -> (error out=w1941:errorcluster)  [unwired: 1 in, 2 out]
      }
      event "Inst_alm_thresh": Value Change {
        n765 = event-data() -> ("NewVal"=w1947:i32)  [unwired: 1 in]
        n766 = Bundle(cluster=T4 {"Message"="", "Message Data"=variant} ("Message Cluster"), "Message"="Inst_alm_thresh", "Message Data"=w1947) -> (w1951:T4)
        n767 = Enqueue Element(queue=w1950, element=w1951, error in (no error)=w1949) -> (error out=w1948:errorcluster)  [unwired: 1 in, 2 out]
      }
      event "3hr_alm_thresh": Value Change {
        n768 = event-data() -> ("NewVal"=w1954:i32)  [unwired: 1 in]
        n769 = Bundle(cluster=T4 {"Message"="", "Message Data"=variant} ("Message Cluster"), "Message"="3hr_alm_thresh", "Message Data"=w1954) -> (w1958:T4)
        n770 = Enqueue Element(queue=w1957, element=w1958, error in (no error)=w1956) -> (error out=w1955:errorcluster)  [unwired: 1 in, 2 out]
      }
      event "Simulate 3hr Average Conc": Value Change {
        n771 = event-data() -> ("NewVal"=w1961:dbl)  [unwired: 1 in]
        n772 = Bundle(cluster=T4 {"Message"="", "Message Data"=variant} ("Message Cluster"), "Message"="Simulate_3hr_av_conc", "Message Data"=w1961) -> (w1965:T4)
        n773 = Enqueue Element(queue=w1964, element=w1965, error in (no error)=w1963) -> (error out=w1962:errorcluster)  [unwired: 1 in, 2 out]
      }
      event "cRIO File IO Stop\n(USB Flash Drive Unmount)": Value Change {
        n774 = event-data() -> ("NewVal"=w1968:bool)  [unwired: 1 in]
        n775 = Bundle(cluster=T4 {"Message"="", "Message Data"=variant} ("Message Cluster"), "Message"="Stop File Write", "Message Data"=w1968) -> (w1972:T4)
        n776 = Enqueue Element(queue=w1971, element=w1972, error in (no error)=w1970) -> (error out=w1969:errorcluster)  [unwired: 1 in, 2 out]
      }
      event "Confirm Flight Number": Value Change {
        n777 = event-data() -> ()  [unwired: 1 in, 5 out]
        n778 = local read "Flight Number"() -> (w1975:string)
        n779 = Bundle(cluster=T4 {"Message"="", "Message Data"=variant} ("Message Cluster"), "Message"="Flight Number", "Message Data"=w1975) -> (w1979:T4)
        n780 = Enqueue Element(queue=w1978, element=w1979, error in (no error)=w1977) -> (error out=w1976:errorcluster)  [unwired: 1 in, 2 out]
      }
    }
    "2BOzone Event error out" <- w1922
  }
  n781 = while {
    tunnel: w23 -> [w1989]
    shift-right: [w1984] -> _
    shift-left: w18 -> [w1986]
    shift-right: [w1982] -> w15
    shift-left: w19 -> [w1988]
    tunnel: w16 -> [w1983]
    stop <- w1982 stop-if-true
    # "2BOzone UI Command Sender"
    n782 = Dequeue Element(queue=w1989, error in (no error)=w1983) -> (element=w1985:T4)  [unwired: 1 in, 3 out]
    n783 = Unbundle By Name(w1985) -> ("Message"=w1987:string)
    n784 = case shown="\"3hr_alm_thresh\"" w1987 {
      tunnel: w1988 -> [w1990 w1994 w2001 w2008 w2015 w2022 w2029 w2036 w2043]
      tunnel: w1986 -> [w1991 w1997 w2004 w2011 w2018 w2025 w2032 w2039 w2046]
      tunnel: w1985 -> [_ w1996 w2003 w2010 w2017 w2024 w2031 w2038 w2045]
      tunnel: [w1990 w1993 w2000 w2007 w2014 w2021 w2028 w2035 w2042] -> w1982
      tunnel: [w1991 w1992 w1999 w2006 w2013 w2020 w2027 w2034 w2041] -> w1984
      frame "False", Default {
      }
      frame "Ambient/Cabin" {
        n785 = shared-variable-write(w1997, w1994, w1996) -> (w1995:refnum<k21>, w1998:errorcluster)  [unwired: 1 in, 1 out]
        n786 = Flush Stream(8:w1998, 11:w1995) -> (0:w1993:errorcluster, 3:w1992:refnum<k21>)  [unwired: 2 in, 1 out]
      }
      frame "Simulate_conc" {
        n787 = shared-variable-write(w2004, w2001, w2003) -> (w2002:refnum<k21>, w2005:errorcluster)  [unwired: 1 in, 1 out]
        n788 = Flush Stream(8:w2005, 11:w2002) -> (0:w2000:errorcluster, 3:w1999:refnum<k21>)  [unwired: 2 in, 1 out]
      }
      frame "Simulate_inst_conc" {
        n789 = shared-variable-write(w2011, w2008, w2010) -> (w2009:refnum<k21>, w2012:errorcluster)  [unwired: 1 in, 1 out]
        n790 = Flush Stream(8:w2012, 11:w2009) -> (0:w2007:errorcluster, 3:w2006:refnum<k21>)  [unwired: 2 in, 1 out]
      }
      frame "Inst_alm_thresh" {
        n791 = shared-variable-write(w2018, w2015, w2017) -> (w2016:refnum<k21>, w2019:errorcluster)  [unwired: 1 in, 1 out]
        n792 = Flush Stream(8:w2019, 11:w2016) -> (0:w2014:errorcluster, 3:w2013:refnum<k21>)  [unwired: 2 in, 1 out]
      }
      frame "3hr_alm_thresh" {
        n793 = shared-variable-write(w2025, w2022, w2024) -> (w2023:refnum<k21>, w2026:errorcluster)  [unwired: 1 in, 1 out]
        n794 = Flush Stream(8:w2026, 11:w2023) -> (0:w2021:errorcluster, 3:w2020:refnum<k21>)  [unwired: 2 in, 1 out]
      }
      frame "Simulate_3hr_av_conc" {
        n795 = shared-variable-write(w2032, w2029, w2031) -> (w2030:refnum<k21>, w2033:errorcluster)  [unwired: 1 in, 1 out]
        n796 = Flush Stream(8:w2033, 11:w2030) -> (0:w2028:errorcluster, 3:w2027:refnum<k21>)  [unwired: 2 in, 1 out]
      }
      frame "Stop File Write" {
        n797 = shared-variable-write(w2039, w2036, w2038) -> (w2037:refnum<k21>, w2040:errorcluster)  [unwired: 1 in, 1 out]
        n798 = Flush Stream(8:w2040, 11:w2037) -> (0:w2035:errorcluster, 3:w2034:refnum<k21>)  [unwired: 2 in, 1 out]
      }
      frame "Flight Number" {
        n799 = shared-variable-write(w2046, w2043, w2045) -> (w2044:refnum<k21>, w2047:errorcluster)  [unwired: 1 in, 1 out]
        n800 = Flush Stream(8:w2047, 11:w2044) -> (0:w2042:errorcluster, 3:w2041:refnum<k21>)  [unwired: 2 in, 1 out]
      }
    }
  }
  "2BOzone command sender error out" <- w15
